vi "Spectrometer.vi"() -> ()   [LabVIEW 2018]
doc: "Demonstrates continuous waveform measurement. Spectrum is displayed in a waveform graph."
uses:
  <vilib>/Analysis/NI_AALBase.lvlib
  <vilib>/Analysis/baseanly.llb/Mean (DBL).vi
  <vilib>/Instr/_visa.llb/VISA Configure Serial Port (Instr).vi
panel:
  out "output cluster":T1={"Temperature Data"={"Bandwidth"=[10, 10, 10], "Bandwidth labels"=["Bandwidth 1-2", "Bandwidth 2-3", "Bandwidth 1-3"], "Color Temperatures"=[[nan], [nan], [nan]], "Wavelength labels"=["Temp1050-1120", "Temp1050-1230", "Temp1120-1230"], "seconds since 1Jan1904"=timestamp(3606762291.6799974 s since 1904-01-01)}, "Vis Data"={{"visible wl array"=array[2028 elements], array[2028 elements]}, {"Vis or NIR"="Visible", "Multiplexer Response"="1", "Wavelength Difference Vis (nm)"=100.0, "Vis Integration Time (ms)"=200, "Normalization path"=path "E:/Materials Testing/Calibration/2017-11-09/Multiplexter.tdms", "Vis background wave"={array[2028 elements], array[2028 elements]}}}, "NIR Data"={{"NIR wl array"=array[512 elements], array[512 elements]}, {"Vis or NIR"="NIR", "Multiplexer Response"="1", "NIR Integration Time (ms)"=50, "Wavelength Difference NIR (nm) "=100.0, "Normalization path"=path "E:/Materials Testing/Calibration/2017-11-09/Multiplexter.tdms", "NIR background wave"={array[512 elements], array[512 elements]}}}}
  out "NIR Data":T2={{"NIR wl array"=array[512 elements], array[512 elements]}, {"Vis or NIR"="NIR", "Multiplexer Response"="1", "NIR Integration Time (ms)"=50, "Wavelength Difference NIR (nm) "=100.0, "Normalization path"=path "E:/Materials Testing/Calibration/2017-11-09/Multiplexter.tdms", "NIR background wave"={array[512 elements], array[512 elements]}}}
  out "Vis Data":T3={{"visible wl array"=array[2028 elements], array[2028 elements]}, {"Vis or NIR"="Visible", "Multiplexer Response"="1", "Wavelength Difference Vis (nm)"=100.0, "Vis Integration Time (ms)"=200, "Normalization path"=path "E:/Materials Testing/Calibration/2017-11-09/Multiplexter.tdms", "Vis background wave"={array[2028 elements], array[2028 elements]}}}
  out "NIR status":bool=TRUE
  out "Vis Status":bool=TRUE
  out "file size":i64
  in  "Save NIR":bool
  in  "Save vis":bool
  in  "Tab Control 2":enum32{"Main", "Extra", "Norm", "Temperature"}(tab)
  out "Norm Visible Intensity":cluster{dbl[], dbl[]}(graph)
  out "Overload vis":bool
  out "Norm NIR Intensity":cluster{dbl[], dbl[]}(graph)
  out "Overload NIR":bool
  in  "Bandwidth 1":i32=10
  in  "Wavelength 1":dbl=1050.0 format="%#_13g"
  out "stddev":dbl=20.177756573412168
  out "Mean":dbl=-49.89258514096029 format="%0.2f"
  out "Temp 1-2":dbl=nan
  in  "Bandwidth 2":i32=10
  in  "Wavelength 2":dbl=1120.0 format="%#_13g"
  out "stddev 2":dbl=26.325405246633235
  out "Mean 2":dbl=-31.365757752015657 format="%0.2f"
  out "Temp 1-3":dbl=nan
  in  "Bandwidth 3":i32=10
  in  "Wavelength 3":dbl=1230.0 format="%#_13g"
  out "Mean 3":dbl=-15.527840110907093 format="%0.2f"
  out "stddev 3":dbl=7.686763202446039
  out "Temp 2-3":dbl=nan
  out "Visible Raw":cluster{dbl[], dbl[]}(graph)
  out "NIR Raw":cluster{dbl[], dbl[]}(graph)
  out "Subtracted NIR":cluster{dbl[], dbl[]}(graph)
  out "Subtracted Avg NIR":dbl=-353.76370072834914 format="%0.2f"
  out "Subtracted Vis":cluster{dbl[], dbl[]}(graph)
  out "Subtracted Avg Vis":dbl=-252.1229874047288 format="%0.2f"
  out "Vis norm wave":cluster{dbl[], dbl[]}(graph)
  out "NIR norm wave":cluster{dbl[], dbl[]}(graph)
  out "NIR background wave":cluster{dbl[], dbl[]}(graph)
  in  "Aquire BG vis":bool
  in  "Reset BG Vis":bool
  in  "Aquire BG NIR":bool
  in  "Reset BG NIR":bool
  out "# averages Vis":i32=10
  out "# averages NIR":i32=43
  out "Vis background wave":cluster{dbl[], dbl[]}(graph)
  in  "Wavelength Difference NIR (nm)":dbl=100.0
  out "Color Temperature NIR":cluster{"wl out":dbl[], "FT":dbl[]}(graph)={"wl out"=array[231 elements], "FT"=[nan, nan, nan, nan, nan, nan, nan, nan, nan, nan, nan, nan, nan, nan, nan, nan, nan, nan, nan, nan, nan, nan, nan, nan, nan, nan, nan, nan, nan, nan, nan, nan, nan, nan, nan, nan, nan, nan, nan, nan, nan, nan, nan, nan, nan, nan, nan, nan, nan, nan, nan, nan, nan, nan, nan, nan, nan, nan, nan, nan, nan, nan, nan, nan, nan, nan, nan, nan, nan, nan, nan, nan, nan, nan, nan, nan, nan, nan, nan, nan, nan, nan, nan, nan, nan, nan, nan, nan, nan, nan, nan, nan, nan, nan, nan, nan, nan, nan, nan, nan, nan, nan, nan, nan, nan, nan, nan, nan, nan, nan, nan, nan, nan, nan, nan, nan, nan, nan, nan, nan, nan, nan, nan, nan, nan, nan, nan, nan, nan, nan, nan, nan, nan, nan, nan, nan, nan, nan, nan, nan, nan, nan, nan, nan, nan, nan, nan, nan, nan, nan, nan, nan, nan, nan, nan, nan, nan, nan, nan, nan, nan, nan, nan, nan, nan, nan, nan, nan, nan, nan, nan, nan, nan, nan, nan, nan, nan, nan, nan, nan, nan, nan, nan, nan, nan, nan, nan, nan, nan, nan, nan, nan, nan, nan, nan, nan, nan, nan, nan, nan, nan, nan, nan, nan, nan, nan, nan, nan, nan, nan, nan, nan, nan, nan, nan, nan, nan, nan, nan, nan, nan, nan, nan, nan, nan, nan, nan, nan, nan, nan, nan]}
  in  "Wavelength Difference Vis (nm)":dbl=100.0
  out "Color Temperature Vis":cluster{"wl out":dbl[], "FT":dbl[]}(graph)
  in  "Tab Control":enum32{"Aquisition", "Setup", "File"}(tab)=enum."Setup"
  in  "Position":i32=1 min=0 max=7
  in  "Multiplexer Command":T4(ring)
  out "Multiplexer Response":string="1"
  in  "Send to multiplexer":bool
  out "NIR aq #":i32=1
  out "vis aq #":i32=1
  in  "save both":bool
  out "MP0 obtained":bool
  out "MP1 obtained":bool
  in  "Stop aquisition":bool
  in  "Multiplexer":refnum<visa-resource-name>="COM7"
  in  "NIR address":refnum<visa-resource-name>="USB0::0x2457::0x1026::NI-VISA-80002::RAW"
  in  "Visible address":refnum<visa-resource-name>="USB0::0x2457::0x101E::NI-VISA-80001::RAW"
  in  "NIR Integration Time (ms)":u32=50
  in  "Vis Integration Time (ms)":u32=200
  in  "set vis aq":i32=50
  in  "set IR aq":i32=100
  in  "Autoswitch":bool
  in  "Use NIR?":bool=TRUE
  in  "Use Vis?":bool=TRUE
  in  "Use MP":bool=TRUE
  in  "Vis every x aquisition":i32=1
  in  "NIR every x aquisition":i32=1
  in  "Mode":T5(ring)
  in  "reset aquisitions":bool
  in  "Cal params":bool
  in  "Clear":bool
  in  "Filename":string="Run1_Spectrometer"
  in  "base path":path=path "E:/Materials Testing"
  out "file path":path=path "E:/Materials Testing/2018-04-16/Run2_Spectrometer.tdms"
  in  "Normalization path":path=path "E:/Materials Testing/Calibration/2017-11-09/Multiplexter.tdms"
  out "Chg vis time":bool
  out "Change NIR time":bool
  out "tdms error out":errorcluster
  out "tdms file out":refnum<k34>
  out "visible wl array":dbl[](array[numeric])=[197.50078789145437, 197.86086398449223, 198.2209166909286, 198.58094600092215, 198.9409519046316, 199.30093439221562, 199.66089345383293, 200.02082907964217, 200.38074125980208, 200.7406299844713, 201.10049524380858, 201.46033702797257, 201.82015532712202, 202.17995013141555, 202.53972143101186, 202.89946921606966, 203.25919347674764, 203.6188942032045, 203.9785713855989, 204.33822501408957, 204.6978550788352, 205.05746156999442, 205.417044477726, 205.77660379218858, 206.13613950354087, 206.49565160194152, 206.85514007754927, 207.21460492052282, 207.5740461210208, 207.93346366920198, 208.292857555225, 208.65222776924855, 209.0115743014313, 209.370897141932, 209.73019628090933, 210.08947170852198, 210.44872341492857, 210.80795139028788, 211.16715562475855, 211.52633610849932, 211.8854928316688, 212.24462578442572, 212.6037349569288, 212.96282033933673, 213.32188192180817, 213.6809196945018, 214.03993364757636, 214.3989237711905, 214.75789005550288, 215.1168324906723, 215.47575106685738, 215.8346457742168, 216.19351660290926, 216.5523635430935, 216.91118658492812, 217.2699857185719, 217.62876093418345, 217.98751222192146, 218.34623957194475, 218.7049429744119, 219.0636224194816, 219.42227789731257, 219.78090939806347, 220.13951691189305, 220.49810042895996, 220.85665993942288, 221.21519543344058, 221.57370690117162, 221.9321943327748, 222.29065771840874, 222.6490970482322, 223.00751231240378, 223.36590350108227, 223.7242706044263, 224.08261361259454, 224.44093251574577, 224.7992273040386, 225.15749796763174, 225.5157444966839, 225.87396688135377, 226.23216511179996, 226.59033917818132, 226.9484890706564, 227.30661477938395, 227.66471629452266, 228.0227936062312, 228.38084670466833, 228.7388755799926, 229.09688022236284, 229.45486062193766, 229.81281676887576, 230.1707486533359, 230.52865626547668, 230.88653959545687, 231.24439863343508, 231.6022333695701, 231.96004379402046, 232.31782989694503, 232.6755916685024, 233.0333290988513, 233.3910421781504, 233.74873089655836, 234.10639524423397, 234.46403521133578, 234.82165078802265, 235.1792419644531, 235.53680873078594, 235.89435107717983, 236.2518689937934, 236.60936247078544, 236.9668314983146, 237.32427606653954, 237.68169616561894, 238.0390917857116, 238.3964629169761, 238.75380954957114, 239.11113167365548, 239.46842927938778, 239.82570235692668, 240.1829508964309, 240.5401748880592, 240.89737432197015, 241.25454918832256, 241.611699477275, 241.96882517898626, 242.325926283615, 242.6830027813199, 243.04005466225968, 243.39708191659298, 243.75408453447852, 244.11106250607497, 244.46801582154106, 244.82494447103548, 245.1818484447169, 245.53872773274398, 245.89558232527546, 246.25241221247003, 246.60921738448633, 246.9659978314831, 247.322753543619, 247.6794845110528, 248.03619072394306, 248.3928721724486, 248.749528846728, 249.10616073694, 249.46276783324333, 249.8193501257966, 250.17590760475855, 250.5324402602879, 250.88894808254327, 251.24543106168338, 251.60188918786693, 251.95832245125263, 252.31473084199914, 252.67111435026513, 253.02747296620936, 253.38380667999044, 253.74011548176713, 254.0963993616981, 254.45265830994202, 254.8088923166576, 255.1651013720035, 255.52128546613844, 255.87744458922117, 256.2335787314102, 256.5896878828644, 256.9457720337424, 257.3018311742029, 257.65786529440453, 258.0138743845061, 258.36985843466624, 258.7258174350435, 259.0817513757968, 259.43766024708475, 259.79354403906603, 260.1494027418993, 260.5052363457432, 260.8610448407566, 261.21682821709805, 261.57258646492625, 261.92831957439995, 262.2840275356779, 262.6397103389185, 262.99536797428084, 263.35100043192335, 263.7066077020047, 264.0621897746837, 264.41774664011905, 264.7732782884694, 265.1287847098934, 265.48426589454976, 265.8397218325972, 266.19515251419443, 266.55055792950014, 266.9059380686729, 267.2612929218716, 267.6166224792547, 267.97192673098107, 268.32720566720934, 268.68245927809824, 269.0376875538064, 269.3928904844925, 269.74806806031535, 270.1032202714335, 270.4583471080056, 270.81344856019064, 271.168524618147, 271.5235752720335, 271.87860051200875, 272.2336003282316, 272.58857471086054, 272.94352365005443, 273.29844713597197, 273.6533451587717, 274.0082177086124, 274.3630647756526, 274.71788635005134, 275.07268242196704, 275.4274529815584, 275.7821980189842, 276.1369175244032, 276.4916114879739, 276.8462798998551, 277.20092275020545, 277.5555400291837, 277.9101317269485, 278.26469783365854, 278.61923833947253, 278.9737532345491, 279.328242509047, 279.682706153125, 280.0371441569416, 280.3915565106556, 280.74594320442577, 281.1003042284106, 281.45463957276894, 281.8089492276594, 282.16323318324083, 282.51749142967174, 282.87172395711076, 283.2259307557168, 283.5801118156484, 283.9342671270643, 284.2883966801232, 284.64250046498387, 284.99657847180487, 285.3506306907448, 285.70465711196255, 286.05865772561685, 286.4126325218662, 286.7665814908693, 287.12050462278506, 287.474401907772, 287.82827333598885, 288.1821188975942, 288.53593858274684, 288.8897323816055, 289.24350028432883, 289.59724228107547, 289.95095836200414, 290.3046485172736, 290.6583127370424, 291.0119510114694, 291.36556333071314, 291.71914968493246, 292.0727100642859, 292.4262444589323, 292.7797528590301, 293.1332352547383, 293.4866916362154, 293.84012199362024, 294.1935263171113, 294.54690459684736, 294.9002568229872, 295.25358298568943, 295.6068830751127, 295.96015708141584, 296.3134049947575, 296.66662680529623, 297.0198225031908, 297.37299207859996, 297.7261355216824, 298.0792528225967, 298.43234397150167, 298.78540895855593, 299.1384477739182, 299.4914604077471, 299.8444468502015, 300.1974070914399, 300.55034112162116, 300.90324893090377, 301.2561305094466, 301.60898584740823, 301.96181493494737, 302.3146177622227, 302.66739431939305, 303.02014459661694, 303.3728685840531, 303.7255662718604, 304.0782376501972, 304.4308827092223, 304.78350143909466, 305.1360938299727, 305.48865987201515, 305.8411995553807, 306.1937128702281, 306.546199806716, 306.89866035500313, 307.25109450524815, 307.60350224760975, 307.9558835722466, 308.30823846931736, 308.6605669289809, 309.0128689413957, 309.3651444967206, 309.71739358511417, 310.06961619673524, 310.42181232174227, 310.77398195029417, 311.1261250725496, 311.4782416786672, 311.83033175880564, 312.18239530312366, 312.53443230177993, 312.88644274493316, 313.238426622742, 313.5903839253652, 313.9423146429613, 314.29421876568927, 314.64609628370755, 314.997947187175, 315.34977146625016, 315.70156911109177, 316.0533401118586, 316.4050844587093, 316.75680214180244, 317.1084931512969, 317.46015747735123, 317.8117951101242, 318.1634060397745, 318.5149902564608, 318.8665477503418, 319.21807851157615, 319.5695825303225, 319.9210597967397, 320.27251030098626, 320.623934033221, 320.9753309836027, 321.32670114228983, 321.67804449944117, 322.02936104521535, 322.3806507697712, 322.7319136632674, 323.0831497158624, 323.4343589177152, 323.7855412589844, 324.13669672982854, 324.48782532040644, 324.83892702087684, 325.1900018213983, 325.5410497121295, 325.89207068322935, 326.24306472485637, 326.5940318271692, 326.94497198032667, 327.2958851744874, 327.6467713998101, 327.9976306464534, 328.3484629045761, 328.6992681643368, 329.05004641589414, 329.400797649407, 329.75152185503396, 330.1022190229337, 330.4528891432649, 330.8035322061862, 331.1541482018565, 331.5047371204343, 331.85529895207833, 332.20583368694736, 332.5563413152, 332.9068218269949, 333.25727521249087, 333.60770146184655, 333.9581005652206, 334.3084725127717, 334.6588172946586, 335.00913490104006, 335.3594253220745, 335.7096885479209, 336.0599245687378, 336.410133374684, 336.7603149559179, 337.11046930259863, 337.4605964048846, 337.8106962529345, 338.16076883690715, 338.5108141469612, 338.8608321732553, 339.21082290594813, 339.5607863351984, 339.9107224511648, 340.26063124400605, 340.6105127038808, 340.96036682094774, 341.31019358536565, 341.6599929872931, 342.0097650168888, 342.3595096643115, 342.70922691971987, 343.05891677327253, 343.4085792151283, 343.7582142354459, 344.10782182438373, 344.4574019721008, 344.8069546687557, 345.1564799045071, 345.50597766951347, 345.85544795393395, 346.204890747927, 346.5543060416512, 346.90369382526535, 347.2530540889282, 347.60238682279845, 347.9516920170346, 348.3009696617955, 348.6502197472398, 348.99944226352625, 349.3486372008134, 349.6978045492601, 350.04694429902503, 350.3960564402667, 350.7451409631439, 351.09419785781546, 351.4432271144399, 351.7922287231759, 352.14120267418235, 352.4901489576177, 352.83906756364075, 353.18795848241024, 353.5368217040848, 353.8856572188231, 354.2344650167838, 354.5832450881258, 354.93199742300754, 355.28072201158784, 355.62941884402534, 355.9780879104788, 356.3267292011068, 356.6753427060681, 357.02392841552137, 357.3724863196254, 357.72101640853873, 358.0695186724201, 358.41799310142824, 358.7664396857219, 359.11485841545954, 359.4632492808001, 359.8116122719022, 360.15994737892447, 360.50825459202554, 360.8565339013643, 361.20478529709936, 361.5530087693893, 361.9012043083929, 362.2493719042689, 362.59751154717594, 362.9456232272726, 363.2937069347179, 363.6417626596701, 363.9897903922882, 364.3377901227308, 364.68576184115653, 365.03370553772413, 365.38162120259227, 365.72950882591977, 366.0773683978652, 366.42519990858716, 366.7730033482445, 367.1207787069959, 367.46852597500003, 367.8162451424154, 368.163936199401, 368.5115991361154, 368.85923394271725, 369.20684060936514, 369.5544191262181, 369.90196948343447, 370.249491671173, 370.5969856795926, 370.94445149885183, 371.29188911910927, 371.6392985305237, 371.9866797232539, 372.3340326874585, 372.6813574132961, 373.02865389092545, 373.3759221105053, 373.7231620621942, 374.070373736151, 374.4175571225344, 374.76471221150297, 375.1118389932154, 375.4589374578304, 375.8060075955068, 376.1530493964031, 376.50006285067803, 376.84704794849046, 377.1940046799989, 377.54093303536206, 377.8878330047386, 378.23470457828734, 378.58154774616685, 378.92836249853576, 379.27514882555306, 379.62190671737716, 379.96863616416687, 380.3153371560808, 380.66200968327774, 381.00865373591637, 381.3552693041552, 381.7018563781531, 382.0484149480688, 382.39494500406084, 382.74144653628804, 383.087919534909, 383.4343639900825, 383.7807798919671, 384.1271672307216, 384.4735259965047, 384.819856179475, 385.1661577697912, 385.5124307576121, 385.85867513309637, 386.20489088640255, 386.5510780076894, 386.8972364871158, 387.24336631484016, 387.5894674810213, 387.93553997581796, 388.2815837893888, 388.62759891189245, 388.97358533348756, 389.31954304433305, 389.66547203458737, 390.0113722944093, 390.35724381395755, 390.7030865833908, 391.04890059286777, 391.394685832547, 391.74044229258743, 392.08616996314754, 392.431868834386, 392.77753889646175, 393.12318013953336, 393.4687925537594, 393.8143761292986, 394.1599308563098, 394.5054567249516, 394.85095372538257, 395.19642184776154, 395.5418610822473, 395.8872714189983, 396.23265284817336, 396.5780053599312, 396.9233289444304, 397.2686235918298, 397.6138892922879, 397.9591260359636, 398.3043338130155, 398.64951261360216, 398.99466242788253, 399.3397832460151, 399.6848750581586, 400.0299378544717, 400.3749716251133, 400.71997636024184, 401.064952050016, 401.4098986845947, 401.7548162541365, 402.0997047488, 402.44456415874396, 402.7893944741272, 403.1341956851083, 403.4789677818458, 403.8237107544987, 404.1684245932255, 404.5131092881849, 404.8577648295356, 405.2023912074364, 405.54698841204583, 405.8915564335226, 406.23609526202546, 406.58060488771315, 406.9250853007443, 407.2695364912775, 407.6139584494717, 407.95835116548534, 408.30271462947724, 408.64704883160596, 408.99135376203037, 409.33562941090906, 409.6798757684007, 410.0240928246641, 410.36828056985786, 410.7124389941406, 411.0565680876711, 411.40066784060815, 411.74473824311025, 412.0887792853361, 412.4327909574446, 412.77677324959427, 413.12072615194376, 413.46464965465185, 413.8085437478773, 414.1524084217787, 414.49624366651466, 414.84004947224406, 415.18382582912545, 415.5275727273176, 415.87129015697917, 416.2149781082689, 416.5586365713454, 416.90226553636734, 417.24586499349346, 417.5894349328825, 417.9329753446931, 418.27648621908395, 418.6199675462138, 418.96341931624124, 419.306841519325, 419.65023414562376, 419.99359718529627, 420.3369306285012, 420.6802344653972, 421.023508686143, 421.3667532808972, 421.70996823981864, 422.0531535530659, 422.3963092107977, 422.73943520317283, 423.08253152034973, 423.4255981524874, 423.76863508974435, 424.1116423222792, 424.4546198402508, 424.7975676338178, 425.1404856931389, 425.4833740083726, 425.8262325696779, 426.16906136721343, 426.51186039113765, 426.8546296316094, 427.19736907878746, 427.5400787228304, 427.88275855389685, 428.2254085621457, 428.56802873773546, 428.9106190708249, 429.2531795515727, 429.5957101701376, 429.9382109166782, 430.2806817813532, 430.6231227543214, 430.96553382574143, 431.3079149857719, 431.65026622457157, 431.9925875322992, 432.3348788991134, 432.6771403151728, 433.01937177063616, 433.3615732556622, 433.7037447604096, 434.045886275037, 434.3879977897032, 434.7300792945668, 435.07213077978645, 435.4141522355209, 435.7561436519289, 436.098105019169, 436.4400363273999, 436.7819375667805, 437.1238087274694, 437.4656497996251, 437.80746077340643, 438.1492416389722, 438.49099238648097, 438.8327130060914, 439.17440348796214, 439.5160638222521, 439.85769399911976, 440.19929400872394, 440.54086384122326, 440.88240348677647, 441.22391293554205, 441.5653921776791, 441.90684120334595, 442.24826000270144, 442.5896485659041, 442.93100688311296, 443.2723349444864, 443.6136327401831, 443.9549002603621, 444.29613749518177, 444.6373444348009, 444.9785210693781, 445.3196673890722, 445.6607833840418, 446.0018690444455, 446.3429243604423, 446.6839493221906, 447.0249439198492, 447.3659081435767, 447.70684198353194, 448.04774542987354, 448.3886184727602, 448.7294611023505, 449.07027330880334, 449.4110550822773, 449.7518064129309, 450.09252729092316, 450.4332177064126, 450.77387764955796, 451.11450711051776, 451.4551060794509, 451.79567454651607, 452.1362125018717, 452.4767199356768, 452.81719683808996, 453.1576431992698, 453.49805900937497, 453.8384442585643, 454.1787989369965, 454.51912303483, 454.8594165422238, 455.19967944933643, 455.53991174632665, 455.88011342335307, 456.2202844705745, 456.5604248781495, 456.9005346362367, 457.24061373499507, 457.58066216458315, 457.9206799151596, 458.260666976883, 458.6006233399123, 458.9405489944061, 459.280443930523, 459.62030813842165, 459.96014160826087, 460.2999443301994, 460.6397162943957, 460.97945749100876, 461.3191679101971, 461.6588475421194, 461.9984963769343, 462.3381144048007, 462.67770161587714, 463.0172580003222, 463.35678354829486, 463.6962782499536, 464.0357420954572, 464.37517507496415, 464.7145771786335, 465.05394839662364, 465.39328871909333, 465.73259813620143, 466.07187663810646, 466.4111242149671, 466.75034085694205, 467.0895265541902, 467.42868129686997, 467.76780507514013, 468.1068978791595, 468.44595969908664, 468.7849905250803, 469.12399034729907, 469.46295915590173, 469.80189694104706, 470.1408036928936, 470.4796794015999, 470.8185240573251, 471.1573376502276, 471.49612017046593, 471.83487160819914, 472.17359195358574, 472.5122811967844, 472.8509393279538, 473.18956633725276, 473.5281622148398, 473.8667269508738, 474.2052605355132, 474.54376295891706, 474.8822342112437, 475.2206742826519, 475.55908316330056, 475.8974608433482, 476.2358073129534, 476.5741225622751, 476.9124065814719, 477.25065936070246, 477.5888808901253, 477.92707115989947, 478.2652301601835, 478.6033578811358, 478.9414543129156, 479.2795194456812, 479.61755326959144, 479.9555557748049, 480.2935269514804, 480.6314667897766, 480.96937527985216, 481.30725241186565, 481.64509817597605, 481.9829125623418, 482.3206955611216, 482.6584471624743, 482.9961673565586, 483.333856133533, 483.6715134835562, 484.0091393967872, 484.3467338633844, 484.68429687350636, 485.02182841731224, 485.3593284849603, 485.6967970666096, 486.0342341524184, 486.37163973254565, 486.7090137971501, 487.04635633639026, 487.38366734042495, 487.72094679941284, 488.05819470351264, 488.39541104288287, 488.73259580768246, 489.06974898807, 489.40687057420405, 489.7439605562435, 490.08101892434706, 490.41804566867324, 490.75504077938075, 491.09200424662845, 491.4289360605749, 491.7658362113788, 492.1027046891989, 492.4395414841938, 492.7763465865223, 493.11311998634295, 493.44986167381455, 493.7865716390959, 494.1232498723454, 494.4598963637219, 494.79651110338415, 495.1330940814908, 495.46964528820035, 495.8061647136718, 496.1426523480638, 496.4791081815348, 496.8155322042436, 497.151924406349, 497.4882847780096, 497.824613309384, 498.1609099906312, 498.49717481190953, 498.833407763378, 499.1696088351949, 499.5057780175193, 499.8419153005097, 500.1780206743248, 500.51409412912346, 500.85013565506415, 501.18614524230577, 501.5221228810067, 501.8580685613259, 502.1939822734221, 502.5298640074538, 502.8657137535797, 503.20153150195864, 503.5373172427492, 503.87307096611, 504.2087926622, 504.54448232117767, 504.88013993320175, 505.2157654884308, 505.5513589770238, 505.8869203891392, 506.22244971493575, 506.5579469445723, 506.8934120682073, 507.2288450759996, 507.56424595810773, 507.8996147046906, 508.2349513059068, 508.5702557519149, 508.9055280328738, 509.24076813894203, 509.57597606027844, 509.91115178704143, 510.2462953093901, 510.5814066174828, 510.91648570147834, 511.25153255153543, 511.5865471578128, 511.9215295104691, 512.256479599663, 512.591397415553, 512.9262829482982, 513.2611361880572, 513.5959571249882, 513.9307457492506, 514.2655020510026, 514.6002260204029, 514.9349176476106, 515.269576922784, 515.604203836082, 515.9387983776631, 516.2733605376862, 516.6078903063099, 516.9423876736927, 517.2768526299936, 517.6112851653712, 517.9456852699841, 518.280052933991, 518.6143881475507, 518.9486909008219, 519.2829611839629, 519.6171989871331, 519.9514043004906, 520.2855771141943, 520.6197174184027, 520.953825203275, 521.2879004589694, 521.6219431756447, 521.9559533434598, 522.2899309525732, 522.6238759931435, 522.9577884553295, 523.29166832929, 523.6255156051835, 523.959330273169, 524.2931123234048, 524.6268617460498, 524.9605785312627, 525.294262669202, 525.6279141500266, 525.9615329638953, 526.2951191009665, 526.6286725513991, 526.9621933053515, 527.2956813529828, 527.6291366844514, 527.962559289916, 528.2959491595356, 528.6293062834684, 528.9626306518735, 529.2959222549093, 529.6291810827348, 529.9624071255084, 530.295600373389, 530.6287608165352, 530.9618884451056, 531.294983249259, 531.628045219154, 531.9610743449496, 532.2940706168041, 532.6270340248764, 532.9599645593252, 533.2928622103091, 533.6257269679866, 533.9585588225167, 534.2913577640583, 534.6241237827694, 534.9568568688093, 535.2895570123364, 535.6222242035095, 535.9548584324872, 536.2874596894284, 536.6200279644914, 536.9525632478354, 537.2850655296186, 537.6175347999999, 537.9499710491383, 538.2823742671917, 538.6147444443196, 538.9470815706804, 539.2793856364327, 539.6116566317352, 539.9438945467468, 540.2760993716258, 540.6082710965313, 540.9404097116218, 541.2725152070559, 541.6045875729926, 541.9366267995902, 542.2686328770076, 542.6006057954036, 542.9325455449366, 543.2644521157656, 543.596325498049, 543.9281656819459, 544.2599726576144, 544.5917464152136, 544.9234869449022, 545.2551942368387, 545.5868682811819, 545.9185090680907, 546.2501165877233, 546.5816908302387, 546.9132317857957, 547.2447394445527, 547.5762137966686, 547.9076548323019, 548.2390625416117, 548.5704369147561, 548.9017779418941, 549.2330856131847, 549.5643599187861, 549.8956008488572, 550.2268083935564, 550.557982543043, 550.8891232874752, 551.2202306170118, 551.5513045218116, 551.8823449920332, 552.2133520178353, 552.5443255893765, 552.8752656968156, 553.2061723303113, 553.5370454800224, 553.8678851361074, 554.198691288725, 554.5294639280339, 554.8602030441929, 555.1909086273606, 555.5215806676957, 555.8522191553569, 556.182824080503, 556.5133954332924, 556.8439332038841, 557.1744373824366, 557.5049079591088, 557.8353449240591, 558.1657482674464, 558.4961179794293, 558.8264540501665, 559.1567564698169, 559.4870252285388, 559.8172603164911, 560.1474617238325, 560.4776294407218, 560.8077634573174, 561.1378637637782, 561.4679303502629, 561.79796320693, 562.1279623239385, 562.4579276914469, 562.7878592996138, 563.117757138598, 563.4476211985583, 563.7774514696533, 564.1072479420415, 564.4370106058819, 564.766739451333, 565.0964344685538, 565.4260956477024, 565.7557229789379, 566.085316452419, 566.4148760583043, 566.7444017867523, 567.0738936279222, 567.4033515719722, 567.7327756090612, 568.0621657293478, 568.3915219229909, 568.720844180149, 569.0501324909808, 569.3793868456451, 569.7086072343004, 570.0377936471054, 570.3669460742192, 570.6960645058, 571.0251489320068, 571.354199342998, 571.6832157289325, 572.012198079969, 572.3411463862662, 572.6700606379826, 572.9989408252771, 573.3277869383085, 573.656598967235, 573.9853769022158, 574.3141207334094, 574.6428304509742, 574.9715060450694, 575.3001475058535, 575.6287548234851, 575.9573279881229, 576.2858669899257, 576.614371819052, 576.9428424656608, 577.2712789199104, 577.5996811719598, 577.9280492119675, 578.2563830300924, 578.5846826164931, 578.9129479613282, 579.2411790547563, 579.5693758869364, 579.897538448027, 580.2256667281869, 580.5537607175745, 580.881820406349, 581.2098457846686, 581.5378368426922, 581.8657935705785, 582.1937159584861, 582.5216039965738, 582.8494576750003, 583.1772769839243, 583.5050619135044, 583.8328124538992, 584.1605285952676, 584.4882103277681, 584.8158576415597, 585.1434705268006, 585.47104897365, 585.7985929722663, 586.1261025128083, 586.4535775854345, 586.7810181803039, 587.108424287575, 587.4357958974065, 587.7631329999571, 588.0904355853854, 588.4177036438505, 588.7449371655104, 589.0721361405243, 589.399300559051, 589.7264304112487, 590.0535256872763, 590.3805863772927, 590.7076124714565, 591.0346039599261, 591.3615608328606, 591.6884830804185, 592.0153706927583, 592.3422236600389, 592.6690419724191, 592.9958256200574, 593.3225745931126, 593.6492888817434, 593.9759684761084, 594.3026133663662, 594.6292235426757, 594.9557989951956, 595.2823397140844, 595.6088456895009, 595.9353169116038, 596.2617533705517, 596.5881550565035, 596.9145219596176, 597.2408540700529, 597.567151377968, 597.8934138735217, 598.2196415468726, 598.5458343881794, 598.8719923876008, 599.1981155352954, 599.5242038214222, 599.8502572361394, 600.1762757696063, 600.502259411981, 600.8282081534223, 601.1541219840893, 601.4800008941403, 601.8058448737343, 602.1316539130297, 602.4574280021853, 602.7831671313596, 603.1088712907117, 603.4345404704001, 603.7601746605832, 604.0857738514202, 604.4113380330695, 604.7368671956897, 605.0623613294396, 605.3878204244782, 605.7132444709637, 606.038633459055, 606.3639873789108, 606.6893062206898, 607.0145899745506, 607.3398386306519, 607.6650521791527, 607.9902306102114, 608.3153739139866, 608.6404820806371, 608.9655551003217, 609.290592963199, 609.6155956594275, 609.9405631791664, 610.2654955125739, 610.590392649809, 610.91525458103, 611.240081296396, 611.5648727860656, 611.8896290401973, 612.2143500489501, 612.5390358024824, 612.8636862909531, 613.1883015045205, 613.5128814333439, 613.8374260675815, 614.1619353973922, 614.4864094129347, 614.8108481043677, 615.1352514618497, 615.4596194755395, 615.783952135596, 616.1082494321777, 616.4325113554431, 616.7567378955513, 617.0809290426607, 617.40508478693, 617.729205118518, 618.0532900275834, 618.3773395042849, 618.7013535387812, 619.0253321212307, 619.3492752417924, 619.673182890625, 619.997055057887, 620.3208917337372, 620.6446929083343, 620.9684585718371, 621.2921887144039, 621.6158833261939, 621.9395423973655, 622.2631659180772, 622.5867538784881, 622.9103062687568, 623.2338230790418, 623.557304299502, 623.8807499202958, 624.2041599315822, 624.5275343235198, 624.8508730862671, 625.1741762099832, 625.4974436848265, 625.8206755009555, 626.1438716485294, 626.4670321177065, 626.7901568986455, 627.1132459815053, 627.4362993564446, 627.7593170136219, 628.0822989431958, 628.4052451353255, 628.7281555801691, 629.0510302678856, 629.3738691886335, 629.6966723325719, 630.019439689859, 630.3421712506537, 630.6648670051148, 630.9875269434009, 631.3101510556708, 631.6327393320827, 631.9552917627958, 632.2778083379688, 632.6002890477602, 632.9227338823287, 633.2451428318329, 633.5675158864319, 633.8898530362837, 634.2121542715477, 634.5344195823824, 634.856648958946, 635.1788423913978, 635.5009998698962, 635.8231213846001, 636.1452069256677, 636.4672564832583, 636.7892700475303, 637.1112476086423, 637.4331891567532, 637.7550946820215, 638.0769641746062, 638.3987976246655, 638.7205950223585, 639.0423563578438, 639.36408162128, 639.6857708028258, 640.00742389264, 640.3290408808813, 640.650621757708, 640.9721665132793, 641.2936751377538, 641.6151476212899, 641.9365839540466, 642.2579841261824, 642.5793481278561, 642.9006759492262, 643.2219675804517, 643.5432230116911, 643.8644422331031, 644.1856252348464, 644.5067720070798, 644.8278825399617, 645.1489568236511, 645.4699948483066, 645.7909966040868, 646.1119620811505, 646.4328912696564, 646.753784159763, 647.0746407416292, 647.3954610054135, 647.7162449412748, 648.0369925393718, 648.357703789863, 648.6783786829071, 648.999017208663, 649.3196193572893, 649.6401851189446, 649.9607144837876, 650.281207441977, 650.6016639836716, 650.92208409903, 651.2424677782109, 651.562815011373, 651.883125788675, 652.2034001002755, 652.5236379363333, 652.8438392870072, 653.1640041424556, 653.4841324928374, 653.8042243283113, 654.124279639036, 654.4442984151698, 654.7642806468718, 655.0842263243009, 655.4041354376151, 655.7240079769737, 656.0438439325351, 656.3636432944581, 656.6834060529012, 657.0031321980235, 657.3228217199833, 657.6424746089393, 657.9620908550505, 658.2816704484753, 658.6012133793727, 658.9207196379009, 659.240189214219, 659.5596220984856, 659.8790182808594, 660.1983777514988, 660.517700500563, 660.8369865182104, 661.1562357945996, 661.4754483198896, 661.7946240842388, 662.113763077806, 662.4328652907498, 662.7519307132291, 663.0709593354024, 663.3899511474284, 663.708906139466, 664.0278243016737, 664.3467056242102, 664.6655500972341, 664.9843577109044, 665.3031284553796, 665.6218623208182, 665.9405592973792, 666.2592193752213, 666.5778425445029, 666.8964287953828, 667.21497811802, 667.5334905025728, 667.8519659391999, 668.1704044180602, 668.4888059293124, 668.8071704631152, 669.1254980096269, 669.4437885590067, 669.762042101413, 670.0802586270046, 670.3984381259401, 670.7165805883783, 671.0346860044777, 671.3527543643974, 671.6707856582956, 671.9887798763313, 672.306737008663, 672.6246570454496, 672.9425399768495, 673.2603857930219, 673.5781944841249, 673.8959660403175, 674.2137004517583, 674.5313977086062, 674.8490578010196, 675.1666807191574, 675.4842664531782, 675.8018149932406, 676.1193263295035, 676.4368004521255, 676.754237351265, 677.0716370170811, 677.3889994397325, 677.7063246093777, 678.0236125161754, 678.3408631502843, 678.6580765018632, 678.9752525610705, 679.2923913180654, 679.6094927630062, 679.9265568860516, 680.2435836773602, 680.5605731270912, 680.8775252254028, 681.1944399624538, 681.5113173284029, 681.828157313409, 682.1449599076304, 682.4617251012262, 682.7784528843548, 683.095143247175, 683.4117961798455, 683.7284116725249, 684.044989715372, 684.3615302985455, 684.678033412204, 684.9944990465062, 685.310927191611, 685.6273178376766, 685.9436709748622, 686.2599865933264, 686.5762646832277, 686.8925052347247, 687.2087082379765, 687.5248736831414, 687.8410015603783, 688.1570918598459, 688.4731445717027, 688.7891596861077, 689.1051371932192, 689.4210770831963, 689.7369793461975, 690.0528439723814, 690.3686709519068, 690.6844602749322, 691.0002119316166, 691.3159259121186, 691.6316022065969, 691.94724080521, 692.2628416981167, 692.5784048754757, 692.8939303274458, 693.2094180441857, 693.5248680158536, 693.840280232609, 694.1556546846099, 694.4709913620153, 694.7862902549839, 695.1015513536743, 695.4167746482453, 695.7319601288555, 696.0471077856635, 696.3622176088281, 696.6772895885082, 696.9923237148621, 697.3073199780488, 697.6222783682267, 697.9371988755547, 698.2520814901915, 698.5669262022958, 698.8817330020261, 699.1965018795412, 699.511232825, 699.8259258285608, 700.1405808803826, 700.4551979706239, 700.7697770894436, 701.0843182270003, 701.3988213734524, 701.713286518959, 702.0277136536786, 702.34210276777, 702.6564538513917, 702.9707668947027, 703.2850418878613, 703.5992788210265, 703.9134776843567, 704.227638468011, 704.5417611621478, 704.8558457569258, 705.1698922425038, 705.4839006090403, 705.7978708466943, 706.1118029456243, 706.425696895989, 706.7395526879471, 707.0533703116571, 707.367149757278, 707.6808910149686, 707.9945940748871, 708.3082589271924, 708.6218855620434, 708.9354739695985, 709.2490241400166, 709.5625360634564, 709.8760097300764, 710.1894451300354, 710.5028422534921, 710.8162010906052, 711.1295216315334, 711.4428038664353, 711.7560477854696, 712.0692533787951, 712.3824206365706, 712.6955495489543, 713.0086401061054, 713.3216922981825, 713.6347061153439, 713.9476815477489, 714.2606185855557, 714.5735172189233, 714.8863774380101, 715.1991992329749, 715.5119825939765, 715.8247275111737, 716.1374339747248, 716.4501019747889, 716.7627315015244, 717.0753225450901, 717.3878750956447, 717.7003891433469, 718.0128646783554, 718.3253016908287, 718.6377001709259, 718.9500601088051, 719.2623814946255, 719.5746643185457, 719.8869085707242, 720.19911424132, 720.5112813204913, 720.8234097983973, 721.1354996651963, 721.4475509110473, 721.7595635261089, 722.0715375005396, 722.3834728244983, 722.6953694881436, 723.0072274816343, 723.319046795129, 723.6308274187863, 723.9425693427651, 724.2542725572239, 724.5659370523216, 724.8775628182166, 725.1891498450678, 725.500698123034, 725.8122076422735, 726.1236783929453, 726.4351103652082, 726.7465035492206, 727.0578579351411, 727.3691735131288, 727.6804502733422, 727.9916882059399, 728.3028873010805, 728.6140475489232, 728.9251689396261, 729.2362514633481, 729.5472951102481, 729.8582998704846, 730.1692657342163, 730.4801926916018, 730.7910807328, 731.1019298479694, 731.4127400272687, 731.7235112608569, 732.0342435388923, 732.3449368515337, 732.6555911889399, 732.9662065412695, 733.2767828986813, 733.5873202513337, 733.8978185893857, 734.208277902996, 734.5186981823231, 734.8290794175257, 735.1394215987626, 735.4497247161926, 735.759988759974, 736.0702137202659, 736.3803995872267, 736.6905463510154, 737.0006540017903, 737.3107225297105, 737.6207519249343, 737.9307421776207, 738.2406932779282, 738.5506052160156, 738.8604779820415, 739.1703115661646, 739.4801059585438, 739.7898611493374, 740.0995771287046, 740.4092538868035, 740.7188914137934, 741.0284896998324, 741.3380487350796, 741.6475685096935, 741.9570490138331, 742.2664902376567, 742.575892171323, 742.885254804991, 743.1945781288192, 743.5038621329661, 743.8131068075909, 744.1223121428519, 744.4314781289079, 744.7406047559174, 745.0496920140395, 745.3587398934326, 745.6677483842552, 745.9767174766665, 746.285647160825, 746.5945374268891, 746.9033882650178, 747.2121996653698, 747.5209716181035, 747.8297041133779, 748.1383971413516, 748.4470506921832, 748.7556647560315, 749.0642393230551, 749.3727743834128, 749.6812699272632, 749.9897259447649, 750.2981424260768, 750.6065193613575, 750.9148567407659, 751.22315455446, 751.5314127925994, 751.8396314453422, 752.1478105028474, 752.4559499552732, 752.7640497927789, 753.0721100055231, 753.3801305836639, 753.6881115173607, 753.9960527967718, 754.3039544120561, 754.611816353372, 754.9196386108785, 755.2274211747341, 755.5351640350976, 755.8428671821276, 756.1505306059828, 756.458154296822, 756.7657382448037, 757.0732824400868, 757.38078687283, 757.6882515331918, 757.9956764113309, 758.3030614974061, 758.6104067815762, 758.9177122539995, 759.2249779048351, 759.5322037242416, 759.8393897023775, 760.1465358294016, 760.4536420954728, 760.7607084907495, 761.0677350053904, 761.3747216295543, 761.6816683533999, 761.988575167086, 762.2954420607709, 762.6022690246136, 762.909056048773, 763.2158031234071, 763.5225102386753, 763.8291773847359, 764.1358045517478, 764.4423917298694, 764.7489389092598, 765.0554460800773, 765.3619132324808, 765.668340356629, 765.9747274426805, 766.281074480794, 766.5873814611282, 766.893648373842, 767.1998752090938, 767.5060619570423, 767.8122086078463, 768.1183151516645, 768.4243815786557, 768.7304078789783, 769.0363940427911, 769.3423400602532, 769.6482459215226, 769.9541116167584, 770.2599371361191, 770.5657224697637, 770.8714676078505, 771.1771725405385, 771.4828372579864, 771.7884617503526, 772.0940460077959, 772.3995900204751, 772.705093778549, 773.0105572721759, 773.3159804915148, 773.6213634267243, 773.9267060679632, 774.2320084053899, 774.5372704291634, 774.8424921294423, 775.1476734963853, 775.4528145201509, 775.7579151908982, 776.0629754987855, 776.3679954339715, 776.672974986615, 776.9779141468749, 777.2828129049097, 777.587671250878, 777.8924891749386, 778.1972666672502, 778.5020037179714, 778.806700317261, 779.1113564552777, 779.41597212218, 779.7205473081268, 780.0250820032768, 780.3295761977885, 780.6340298818207, 780.9384430455322, 781.2428156790813, 781.5471477726272, 781.8514393163284, 782.1556903003434, 782.4599007148312, 782.7640705499502, 783.0681997958593, 783.3722884427171, 783.6763364806824, 783.9803438999136, 784.2843106905698, 784.5882368428094, 784.892122346791, 785.1959671926736, 785.4997713706158, 785.8035348707763, 786.1072576833136, 786.4109397983865, 786.7145812061538, 787.0181818967741, 787.321741860406, 787.6252610872084, 787.9287395673399, 788.2321772909589, 788.5355742482247, 788.8389304292955, 789.1422458243302, 789.4455204234872, 789.7487542169257, 790.051947194804, 790.355099347281, 790.6582106645152, 790.9612811366654, 791.2643107538904, 791.5672995063485, 791.8702473841989, 792.1731543776, 792.4760204767103, 792.778845671689, 793.0816299526946, 793.3843733098855, 793.6870757334207, 793.9897372134587, 794.2923577401584, 794.5949373036783, 794.8974758941772, 795.1999735018138, 795.5024301167467, 795.8048457291346, 796.1072203291362, 796.4095539069104, 796.7118464526155, 797.0140979564105, 797.316308408454, 797.6184777989047, 797.9206061179212, 798.2226933556623, 798.5247395022868, 798.8267445479531, 799.12870848282, 799.4306312970463, 799.7325129807906, 800.0343535242115, 800.336152917468, 800.6379111507184, 800.9396282141219, 801.2413040978365, 801.5429387920215, 801.8445322868353, 802.1460845724366, 802.447595638984, 802.7490654766367, 803.0504940755528, 803.3518814258912, 803.6532275178106, 803.9545323414696, 804.2557958870271, 804.5570181446417, 804.8581991044721, 805.1593387566768, 805.4604370914146, 805.7614940988444, 806.0625097691247, 806.3634840924143, 806.6644170588717, 806.9653086586557, 807.266158881925, 807.5669677188381, 807.8677351595542, 808.1684611942316, 808.4691458130288, 808.7697890061049, 809.0703907636184, 809.3709510757282, 809.6714699325926, 809.9719473243706, 810.2723832412207, 810.5727776733019, 810.8731306107724, 811.1734420437914, 811.4737119625173, 811.7739403571087, 812.0741272177246, 812.3742725345235, 812.6743762976643, 812.9744384973052, 813.2744591236053, 813.5744381667233, 813.8743756168177, 814.1742714640474, 814.4741256985708, 814.7739383105468, 815.073709290134, 815.3734386274914, 815.6731263127772, 815.9727723361505, 816.2723766877696, 816.5719393577934, 816.8714603363808, 817.17093961369, 817.4703771798802, 817.7697730251099, 818.0691271395377, 818.3684395133223, 818.6677101366224, 818.9669389995969, 819.2661260924041, 819.565271405203, 819.8643749281524, 820.1634366514105, 820.4624565651363, 820.7614346594887, 821.0603709246261, 821.3592653507071, 821.6581179278908, 821.9569286463354, 822.2556974962, 822.5544244676429, 822.8531095508232, 823.1517527358993, 823.45035401303, 823.7489133723742, 824.0474308040901, 824.3459062983369, 824.6443398452728, 824.942731435057, 825.2410810578477, 825.539388703804, 825.8376543630843, 826.1358780258474, 826.4340596822522, 826.732199322457, 827.0302969366207, 827.328352514902, 827.6263660474597, 827.9243375244522, 828.2222669360383, 828.5201542723769, 828.8179995236263, 829.1158026799457, 829.4135637314934, 829.7112826684282, 830.0089594809086, 830.3065941590936, 830.6041866931419, 830.9017370732118, 831.1992452894625, 831.4967113320524, 831.7941351911403, 832.0915168568846, 832.3888563194444, 832.6861535689782, 832.9834085956446, 833.2806213896024, 833.5777919410103, 833.874920240027, 834.1720062768111, 834.4690500415214, 834.7660515243166, 835.0630107153553, 835.3599276047961, 835.656802182798, 835.9536344395194, 836.2504243651191, 836.5471719497558, 836.8438771835882, 837.140540056775, 837.4371605594747, 837.7337386818464, 838.0302744140483, 838.3267677462394, 838.6232186685784, 838.919627171224, 839.2159932443346, 839.5123168780691, 839.8085980625863, 840.1048367880447, 840.4010330446031, 840.6971868224201, 840.9932981116547, 841.2893669024651, 841.5853931850103, 841.8813769494488, 842.1773181859396, 842.473216884641, 842.7690730357122, 843.0648866293113, 843.3606576555975, 843.6563861047291, 843.9520719668649, 844.247715232164, 844.5433158907844, 844.8388739328851, 845.1343893486251, 845.4298621281625, 845.7252922616564, 846.0206797392655, 846.3160245511484, 846.6113266874638, 846.9065861383701, 847.2018028940264, 847.4969769445914, 847.7921082802234, 848.0871968910815, 848.3822427673242, 848.6772458991103, 848.9722062765981, 849.2671238899468, 849.5619987293148, 849.8568307848609, 850.1516200467439, 850.4463665051222, 850.7410701501547, 851.035730972, 851.3303489608169, 851.624924106764, 851.9194564, 852.2139458306835, 852.5083923889734, 852.8027960650282, 853.0971568490068, 853.3914747310677, 853.6857497013696, 853.9799817500714, 854.2741708673313, 854.5683170433086, 854.8624202681618, 855.1564805320493, 855.45049782513, 855.7444721375629, 856.0384034595061, 856.3322917811184, 856.626137092559, 856.9199393839862, 857.2136986455585, 857.5074148674352, 857.8010880397744, 858.094718152735, 858.3883051964757, 858.6818491611554, 858.9753500369324, 859.2688078139655, 859.5622224824136, 859.8555940324353, 860.1489224541893, 860.4422077378341, 860.7354498735285, 861.0286488514313, 861.3218046617011, 861.6149172944966, 861.9079867399766, 862.2010129882997, 862.4939960296243, 862.7869358541096, 863.0798324519142, 863.3726858131964, 863.6654959281152, 863.9582627868292, 864.2509863794972, 864.5436666962777, 864.8363037273297, 865.1288974628114, 865.421447892882, 865.7139550077]
  out "NIR wl array":dbl[](array[numeric])=[890.92688, 894.2151612831569, 897.503264932628, 900.7911909484129, 904.0789393305121, 907.366510078925, 910.653903193652, 913.941118674693, 917.2281565220479, 920.515016735717, 923.8016993156999, 927.088204261997, 930.374531574608, 933.660681253533, 936.9466532987719, 940.2324477103249, 943.518064488192, 946.803503632373, 950.088765142868, 953.373849019677, 956.6587552627999, 959.943483872237, 963.2280348479879, 966.5124081900531, 969.796603898432, 973.0806219731251, 976.3644624141319, 979.6481252214529, 982.931610395088, 986.214917935037, 989.4980478413, 992.781000113877, 996.063774752768, 999.346371757973, 1002.6287911294919, 1005.911032867325, 1009.193096971472, 1012.474983441933, 1015.756692278708, 1019.038223481797, 1022.3195770512, 1025.6007529869169, 1028.881751288948, 1032.162571957293, 1035.443214991952, 1038.723680392925, 1042.003968160212, 1045.2840782938129, 1048.564010793728, 1051.843765659957, 1055.1233428925, 1058.402742491357, 1061.681964456528, 1064.961008788013, 1068.2398754858118, 1071.518564549925, 1074.797075980352, 1078.075409777093, 1081.353565940148, 1084.631544469517, 1087.9093453652001, 1091.1869686271968, 1094.464414255508, 1097.741682250133, 1101.018772611072, 1104.295685338325, 1107.572420431892, 1110.848977891773, 1114.125357717968, 1117.4015599104769, 1120.6775844693, 1123.953431394437, 1127.229100685888, 1130.504592343653, 1133.779906367732, 1137.055042758125, 1140.330001514832, 1143.604782637853, 1146.8793861271881, 1150.153811982837, 1153.4280602048, 1156.7021307930768, 1159.9760237476678, 1163.249739068573, 1166.523276755792, 1169.796636809325, 1173.069819229172, 1176.342824015333, 1179.6156511678078, 1182.888300686597, 1186.1607725717, 1189.433066823117, 1192.705183440848, 1195.977122424893, 1199.248883775252, 1202.5204674919248, 1205.791873574912, 1209.0631020242129, 1212.334152839828, 1215.605026021757, 1218.87572157, 1222.146239484557, 1225.4165797654277, 1228.6867424126128, 1231.956727426112, 1235.226534805925, 1238.4961645520518, 1241.7656166644929, 1245.034891143248, 1248.3039879883167, 1251.5729071997, 1254.841648777397, 1258.110212721408, 1261.3785990317328, 1264.6468077083719, 1267.914838751325, 1271.1826921605918, 1274.4503679361728, 1277.717866078068, 1280.985186586277, 1284.2523294608, 1287.519294701637, 1290.786082308788, 1294.0526922822528, 1297.319124622032, 1300.585379328125, 1303.851456400532, 1307.117355839253, 1310.383077644288, 1313.648621815637, 1316.9139883532998, 1320.179177257277, 1323.444188527568, 1326.7090221641731, 1329.973678167092, 1333.238156536325, 1336.5024572718721, 1339.766580373733, 1343.030525841908, 1346.294293676397, 1349.5578838772, 1352.8212964443169, 1356.084531377748, 1359.3475886774931, 1362.610468343552, 1365.873170375925, 1369.135694774612, 1372.3980415396131, 1375.6602106709279, 1378.922202168557, 1382.1840160325, 1385.445652262757, 1388.707110859328, 1391.968391822213, 1395.229495151412, 1398.490420846925, 1401.7511689087519, 1405.0117393368928, 1408.272132131348, 1411.532347292117, 1414.7923848192, 1418.052244712597, 1421.311926972308, 1424.571431598333, 1427.8307585906718, 1431.089907949325, 1434.348879674292, 1437.607673765573, 1440.866290223168, 1444.124729047077, 1447.3829902373, 1450.6410737938368, 1453.8989797166878, 1457.156708005853, 1460.414258661332, 1463.671631683125, 1466.928827071232, 1470.185844825653, 1473.4426849463878, 1476.699347433437, 1479.9558322868, 1483.2121395064771, 1486.468269092468, 1489.724221044773, 1492.979995363392, 1496.2355920483249, 1499.491011099572, 1502.746252517133, 1506.001316301008, 1509.2562024511972, 1512.5109109676998, 1515.765441850517, 1519.0197950996478, 1522.273970715093, 1525.527968696852, 1528.781789044925, 1532.0354317593121, 1535.288896840013, 1538.542184287028, 1541.7952941003568, 1545.0482262799999, 1548.300980825957, 1551.553557738228, 1554.8059570168132, 1558.058178661712, 1561.3102226729247, 1564.562089050452, 1567.813777794293, 1571.065288904448, 1574.3166223809171, 1577.5677782237, 1580.818756432797, 1584.0695570082078, 1587.320179949933, 1590.5706252579719, 1593.820892932325, 1597.070982972992, 1600.320895379973, 1603.570630153268, 1606.8201872928769, 1610.0695667987998, 1613.3187686710369, 1616.567792909588, 1619.816639514453, 1623.065308485632, 1626.313799823125, 1629.5621135269319, 1632.810249597053, 1636.058208033488, 1639.305988836237, 1642.5535920053, 1645.8010175406769, 1649.048265442368, 1652.295335710373, 1655.542228344692, 1658.788943345325, 1662.035480712272, 1665.2818404455331, 1668.528022545108, 1671.7740270109969, 1675.0198538431998, 1678.2655030417168, 1681.510974606548, 1684.756268537693, 1688.001384835152, 1691.246323498925, 1694.491084529012, 1697.7356679254128, 1700.980073688128, 1704.2243018171569, 1707.4683523125, 1710.712225174157, 1713.955920402128, 1717.199437996413, 1720.442777957012, 1723.685940283925, 1726.9289249771518, 1730.171732036693, 1733.4143614625482, 1736.656813254717, 1739.8990874132, 1743.1411839379969, 1746.3831028291079, 1749.624844086533, 1752.866407710272, 1756.1077937003251, 1759.349002056692, 1762.590032779373, 1765.830885868368, 1769.0715613236769, 1772.3120591453, 1775.552379333237, 1778.7925218874882, 1782.032486808053, 1785.272274094932, 1788.5118837481248, 1791.751315767632, 1794.990570153453, 1798.229646905588, 1801.468546024037, 1804.7072675088, 1807.945811359877, 1811.1841775772677, 1814.4223661609728, 1817.660377110992, 1820.898210427325, 1824.135866109972, 1827.373344158933, 1830.610644574208, 1833.8477673557968, 1837.0847125036998, 1840.3214800179169, 1843.5580698984481, 1846.7944821452932, 1850.030716758452, 1853.2667737379247, 1856.502653083712, 1859.738354795813, 1862.973878874228, 1866.2092253189571, 1869.44439413, 1872.679385307357, 1875.9141988510278, 1879.148834761013, 1882.383293037312, 1885.617573679925, 1888.851676688852, 1892.085602064093, 1895.319349805648, 1898.5529199135167, 1901.7863123876998, 1905.019527228197, 1908.252564435008, 1911.4854240081331, 1914.718105947572, 1917.9506102533248, 1921.182936925392, 1924.4150859637728, 1927.6470573684678, 1930.878851139477, 1934.1104672768001, 1937.341905780437, 1940.573166650388, 1943.804249886653, 1947.0351554892318, 1950.265883458125, 1953.496433793332, 1956.7268064948528, 1959.957001562688, 1963.187018996837, 1966.4168587973, 1969.646520964077, 1972.8760054971679, 1976.105312396573, 1979.3344416622917, 1982.563393294325, 1985.792167292672, 1989.020763657333, 1992.2491823883079, 1995.477423485597, 1998.7054869492, 2001.9333727791168, 2005.1610809753479, 2008.388611537893, 2011.615964466752, 2014.843139761925, 2018.070137423412, 2021.296957451213, 2024.523599845328, 2027.750064605757, 2030.9763517325, 2034.202461225557, 2037.4283930849278, 2040.6541473106129, 2043.879723902612, 2047.1051228609247, 2050.330344185552, 2053.5553878764927, 2056.7802539337476, 2060.004942357317, 2063.2294531472, 2066.453786303397, 2069.677941825908, 2072.901919714733, 2076.125719969872, 2079.349342591325, 2082.5727875790917, 2085.796054933173, 2089.019144653568, 2092.2420567402764, 2095.4647911933, 2098.687348012637, 2101.909727198288, 2105.131928750253, 2108.3539526685317, 2111.575798953125, 2114.797467604032, 2118.018958621253, 2121.240272004788, 2124.4614077546366, 2127.6823658708, 2130.903146353277, 2134.123749202068, 2137.344174417173, 2140.5644219985916, 2143.7844919463246, 2147.004384260372, 2150.224098940733, 2153.443635987408, 2156.662995400397, 2159.8821771797, 2163.101181325317, 2166.3200078372483, 2169.538656715493, 2172.757127960052, 2175.975421570925, 2179.193537548112, 2182.4114758916126, 2185.6292366014277, 2188.8468196775566, 2192.0642251199997, 2195.281452928757, 2198.498503103828, 2201.715375645213, 2204.932070552912, 2208.148587826925, 2211.364927467252, 2214.581089473893, 2217.797073846848, 2221.012880586117, 2224.2285096916994, 2227.4439611635967, 2230.6592350018077, 2233.874331206333, 2237.089249777172, 2240.3039907143248, 2243.5185540177918, 2246.732939687573, 2249.947147723668, 2253.161178126077, 2256.3750308948, 2259.588706029837, 2262.802203531188, 2266.015523398853, 2269.2286656328315, 2272.4416302331247, 2275.6544171997316, 2278.8670265326527, 2282.0794582318877, 2285.291712297437, 2288.5037887293, 2291.7156875274773, 2294.927408691968, 2298.1389522227732, 2301.350318119892, 2304.5615063833247, 2307.772517013072, 2310.983350009133, 2314.1940053715075, 2317.4044831001966, 2320.6147831952, 2323.824905656517, 2327.0348504841477, 2330.2446176780927, 2333.454207238352, 2336.663619164925, 2339.872853457812, 2343.081910117013, 2346.290789142528, 2349.499490534357, 2352.7080142925, 2355.916360416957, 2359.124528907728, 2362.332519764813, 2365.540332988212, 2368.747968577925, 2371.955426533952, 2375.162706856293, 2378.369809544948, 2381.576734599917, 2384.7834820212, 2387.990051808797, 2391.1964439627077, 2394.402658482933, 2397.608695369472, 2400.814554622325, 2404.0202362414916, 2407.225740226973, 2410.431066578768, 2413.636215296877, 2416.8411863813, 2420.045979832037, 2423.250595649088, 2426.455033832453, 2429.659294382132, 2432.863377298125, 2436.0672825804318, 2439.271010229053, 2442.474560243988, 2445.677932625237, 2448.8811273727997, 2452.084144486677, 2455.286983966868, 2458.489645813373, 2461.692130026192, 2464.894436605325, 2468.096565550772, 2471.2985168625332, 2474.500290540608, 2477.7018865849973, 2480.9033049956997, 2484.104545772717, 2487.305608916048, 2490.5064944256924, 2493.7072023016517, 2496.907732543925, 2500.1080851525116, 2503.3082601274127, 2506.508257468628, 2509.708077176157, 2512.90771925, 2516.107183690157, 2519.306470496628, 2522.5055796694132, 2525.704511208512, 2528.903265113925, 2532.101841385652, 2535.3002400236924, 2538.4984610280476, 2541.6965043987166, 2544.8943701357, 2548.0920582389967]
  in  "Stop":bool
  # "Fix multiplexer glitch\nsend notification button"
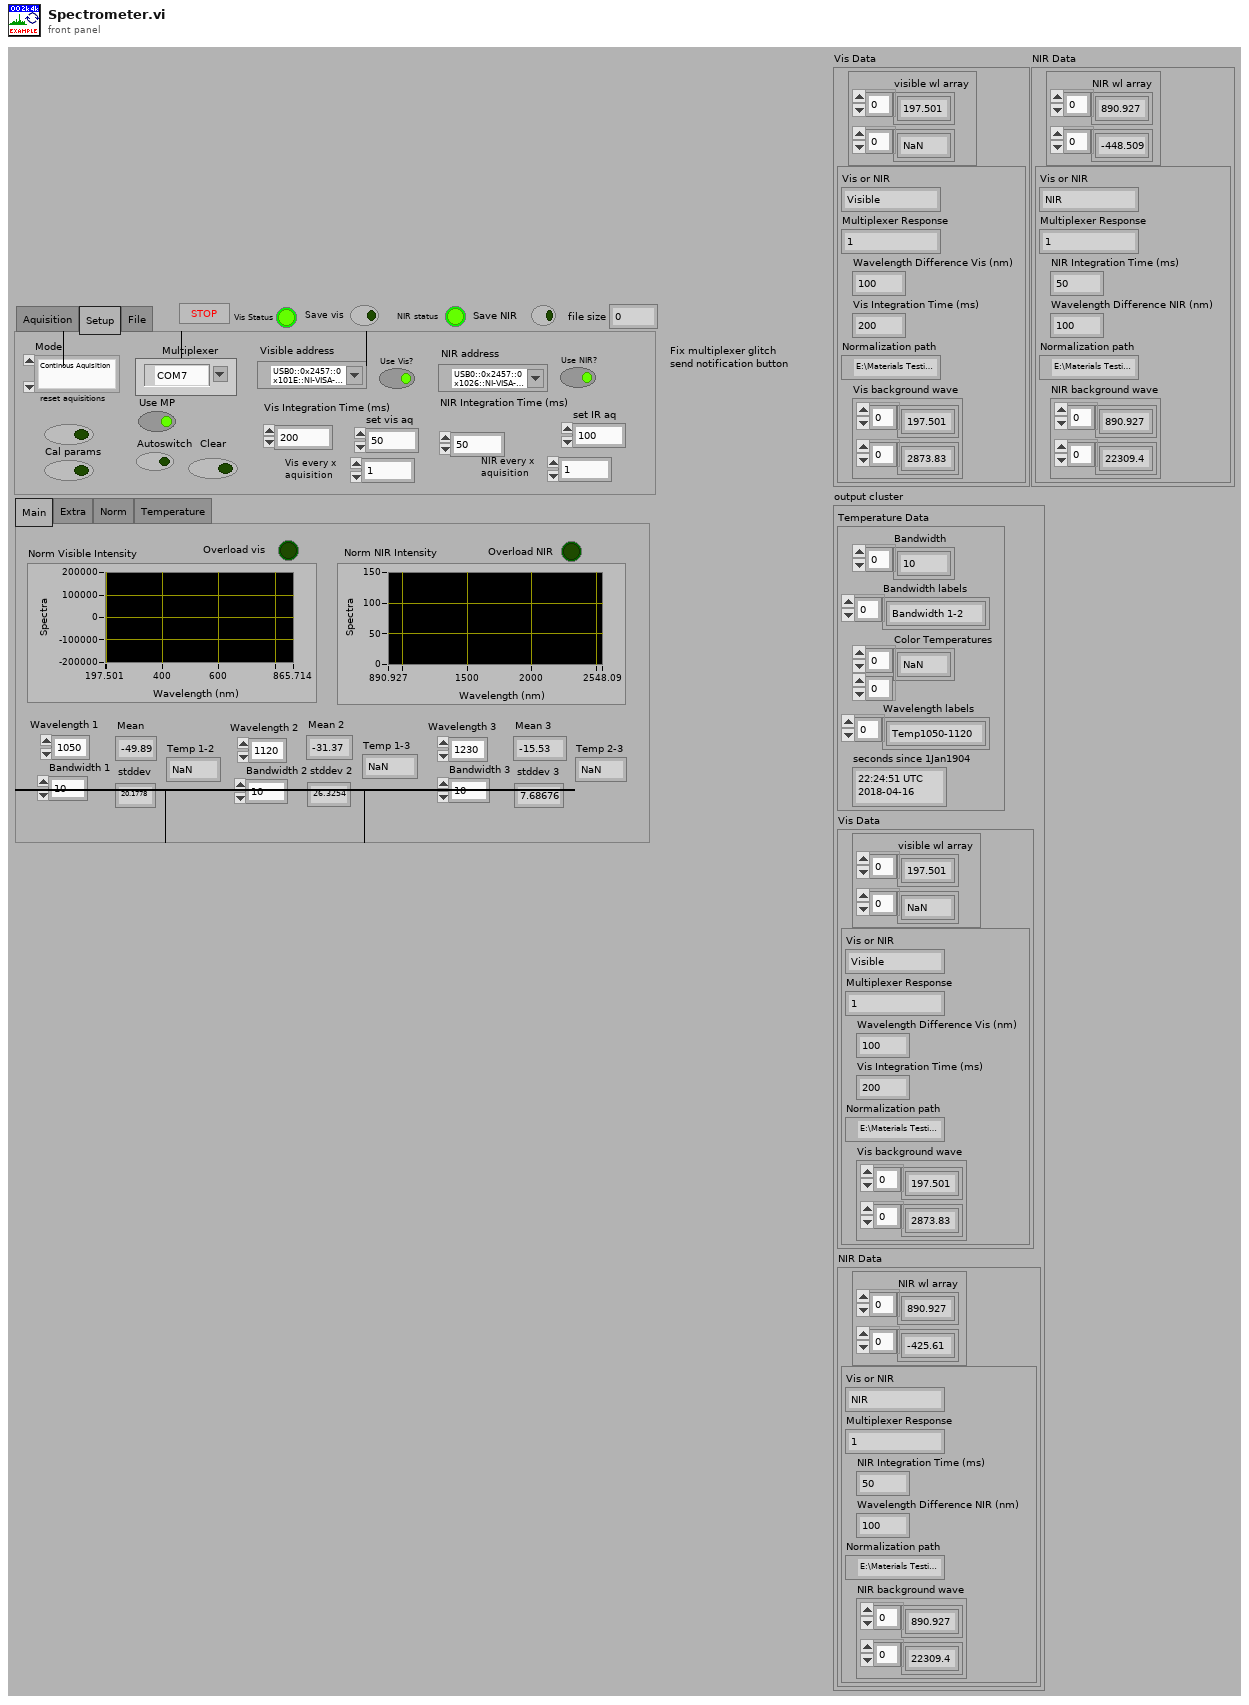
[diagram p1: front panel]
types:
  T1 = cluster{"Temperature Data":cluster{"Bandwidth":i32[], "Bandwidth labels":string[], "Color Temperatures":dbl[][], "Wavelength labels":string[], "seconds since 1Jan1904":timestamp}, "Vis Data":cluster{cluster{"visible wl array":dbl[], dbl[]}, cluster{"Vis or NIR":string, "Multiplexer Response":string, "Wavelength Difference Vis (nm)":dbl, "Vis Integration Time (ms)":u32, "Normalization path":path, "Vis background wave":cluster{dbl[], dbl[]}}}, "NIR Data":cluster{cluster{"NIR wl array":dbl[], dbl[]}, cluster{"Vis or NIR":string, "Multiplexer Response":string, "NIR Integration Time (ms)":u32, "Wavelength Difference NIR (nm) ":dbl, "Normalization path":path, "NIR background wave":cluster{dbl[], dbl[]}}}}
  T2 = cluster{cluster{"NIR wl array":dbl[], dbl[]}, cluster{"Vis or NIR":string, "Multiplexer Response":string, "NIR Integration Time (ms)":u32, "Wavelength Difference NIR (nm) ":dbl, "Normalization path":path, "NIR background wave":cluster{dbl[], dbl[]}}}
  T3 = cluster{cluster{"visible wl array":dbl[], dbl[]}, cluster{"Vis or NIR":string, "Multiplexer Response":string, "Wavelength Difference Vis (nm)":dbl, "Vis Integration Time (ms)":u32, "Normalization path":path, "Vis background wave":cluster{dbl[], dbl[]}}}
  T4 = enum16{"Move position", "Get Status", "Get Program"}
  T5 = enum16{"Continous Aquisition", "Single Aquisition", "Cont switch"}
  T6 = cluster{"Bandwidth":i32[], "Bandwidth labels":string[], "Color Temperatures":dbl[][], "Wavelength labels":string[], "seconds since 1Jan1904":timestamp}
  T7 = cluster{"baud rate":u32, "data bits":u16, "parity":enum16{"None", "Odd", "Even", "Mark", "Space"}, "stop bits":u16, "flow control":u16}
  T8 = cluster{"NIR wl array":dbl[], "Spectrum by Pixel Number":dbl[]}
  T9 = cluster{"Vis or NIR":string, "Multiplexer Response":string, "NIR Integration Time (ms)":u32, "Wavelength Difference NIR (nm) ":dbl, "Normalization path":path, "NIR background wave":cluster{dbl[], dbl[]}}
  T10 = cluster{"visible wl array":dbl[], "Spectrum by Pixel Number":dbl[]}
  T11 = cluster{"Vis or NIR":string, "Multiplexer Response":string, "Wavelength Difference Vis (nm)":dbl, "Vis Integration Time (ms)":u32, "Normalization path":path, "Vis background wave":cluster{dbl[], dbl[]}}
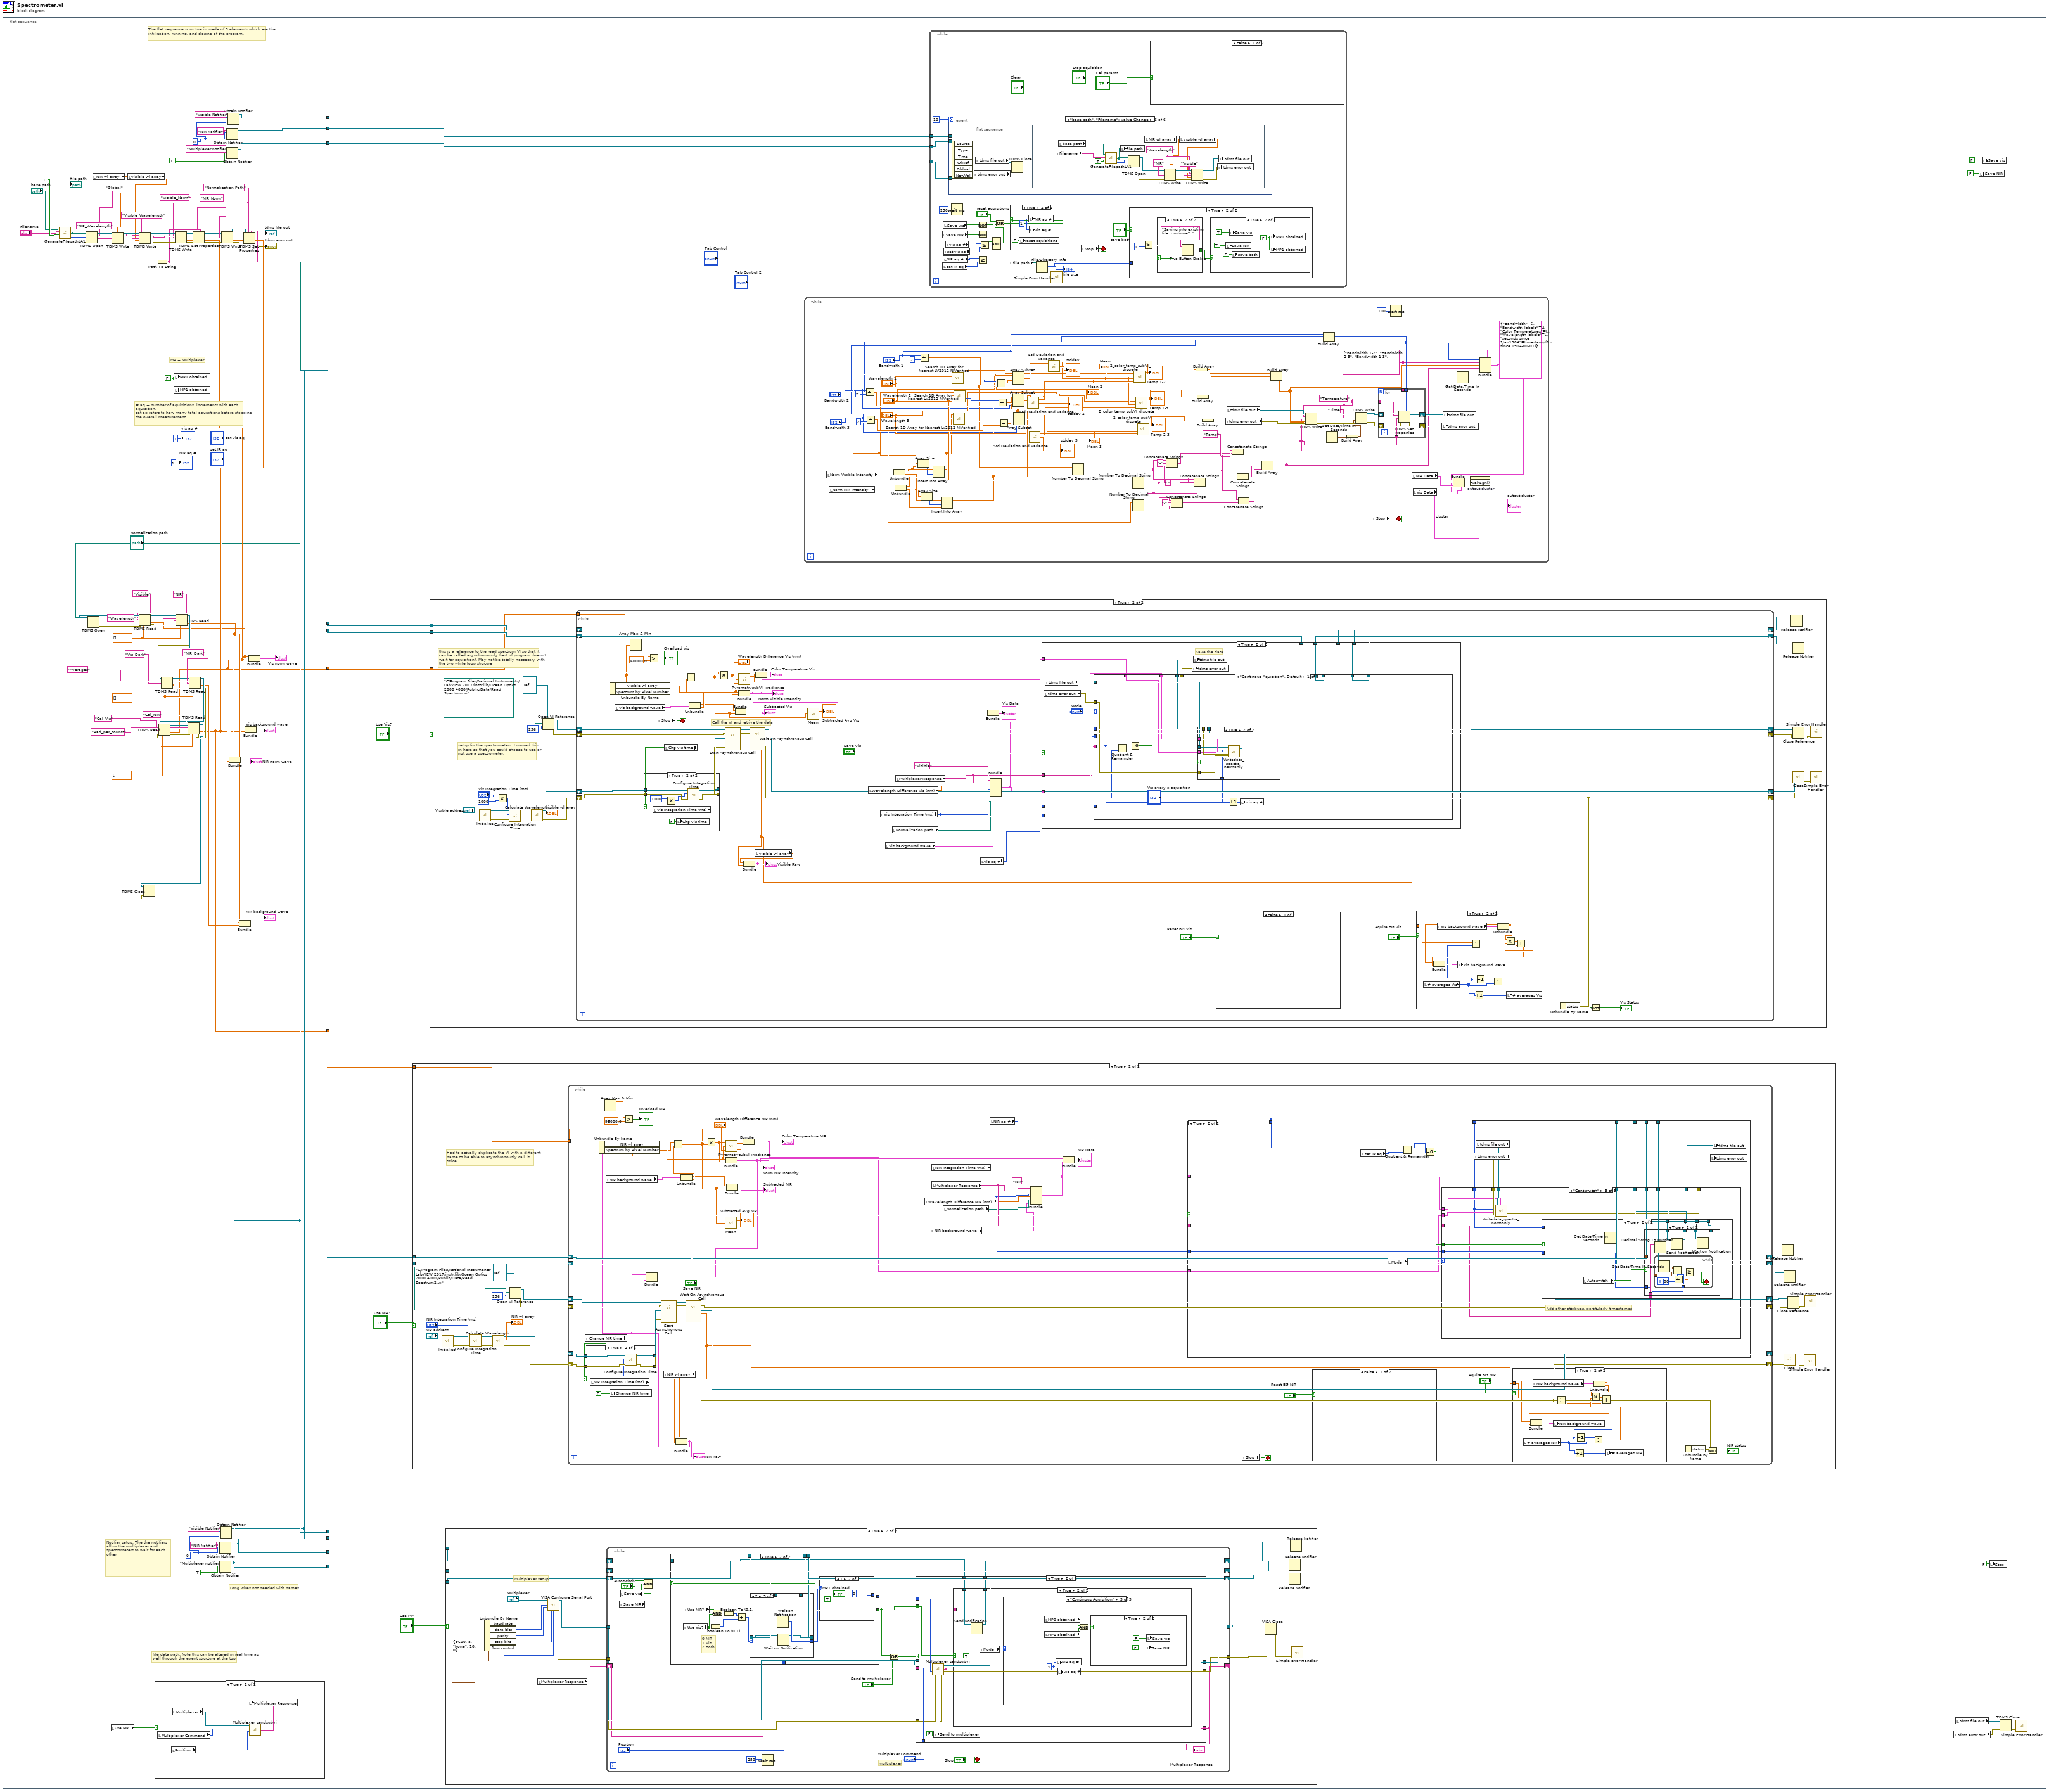
[diagram p0: block diagram]
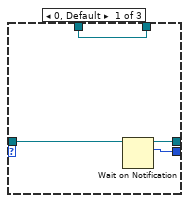
[diagram p5: hidden frame]
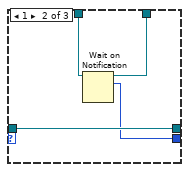
[diagram p6: hidden frame]
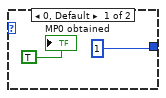
[diagram p7: hidden frame]
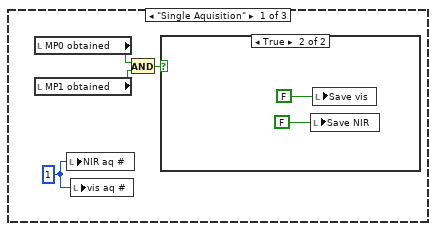
[diagram p10: hidden frame]
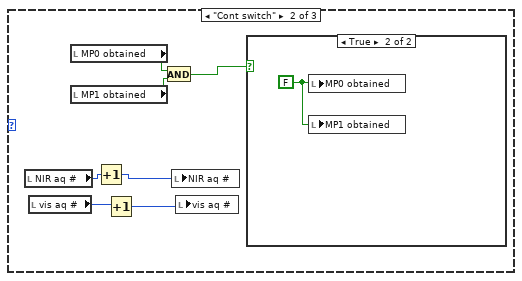
[diagram p12: hidden frame]
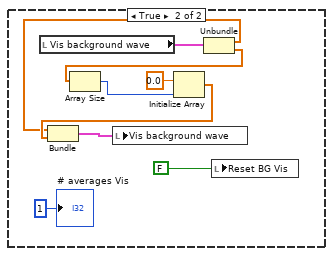
[diagram p17: hidden frame]
diagram:
  n1 = flat-sequence {
    tunnel: [w91] -> w12
    tunnel: [w90] -> w11
    tunnel: [w92] -> w10
    tunnel: [w92] -> w9
    tunnel: [w92] -> w8
    tunnel: [w91] -> w7
    tunnel: [w90] -> w6
    tunnel: [w42] -> w5
    tunnel: [w41] -> w4
    tunnel: [w48] -> w3
    tunnel: [w47] -> w2
    tunnel: [w46] -> w1
    tunnel: w12 -> [w124]
    tunnel: w11 -> [w119]
    tunnel: w10 -> [w120]
    tunnel: w9 -> [w123]
    tunnel: w8 -> [w118]
    tunnel: w7 -> [w121]
    tunnel: w6 -> [w122]
    tunnel: w5 -> [w114]
    tunnel: w4 -> [w113]
    tunnel: w3 -> [w112]
    tunnel: w2 -> [w111]
    tunnel: w1 -> [w110]
    frame #0 {
      w22 = "Normalization Path" ("group name in (Untitled)")
      w52 = 0
      w64 = dbl[] []
      w65 = dbl[] []
      w66 = dbl[] []
      w87 = FALSE ("save both")
      w89 = 0
      # "Long wires not needed with names"
      # "Notifier setup. The the notifiers allow the multiplexer and spectrometers to wait for each other"
      # "file data path. Note this can be altered in real time as well through the event structure at the top"
      # "# aq = number of aquisitions. increments with each aquisition.\nset aq refers to how many total aquisitions before stopping the overall measurement."
      # "MP = Multiplexer"
      # "The flat sequence scructure is made of 3 elements which are the intilization, running, and closing of the program."
      n2 = call "GenerateFilepathLA1.vi"("Auto Date folder"=TRUE, "Filename"="Filename", "base path"="base path") -> ("Numeric"=w14:i32, "file path"=w13:path)  [unwired: 1 in, 1 out]
      "file path" <- w13
      n3 = TDMS Open(10:w14, 11:w13) -> (0:w97:errorcluster, 3:w98:refnum<k34>)  [unwired: 5 in]
      n4 = TDMS Open(11:"Normalization path") -> (0:w83:errorcluster, 3:w84:refnum<k34>)  [unwired: 6 in]
      n5 = local read "NIR wl array"() -> (w99:dbl[])
      n6 = local read "Use MP"() -> (w45:bool)
      n7 = TDMS Write(0:w98, 5:"Global" ("group name in (Untitled)"), 7:"NIR_Wavelength" ("group name in (Untitled)"), 9:w99, 11:w97) -> (4:w102:refnum<k34>, 6:w38:string, 15:w103:errorcluster)  [unwired: 1 in, 1 out]
      n8 = local read "visible wl array"() -> (w96:dbl[])
      n9 = TDMS Write(0:w102, 5:w38, 7:"Visible_Wavelength" ("group name in (Untitled)"), 9:w96, 11:w103) -> (4:w44:refnum<k34>, 6:w39:string, 15:w43:errorcluster)  [unwired: 1 in, 1 out]
      n10 = TDMS Read(0:w84, 5:"Wavelength" ("group name in"), 7:"Visible", 11:w83, 12:w66) -> (4:w79:refnum<k34>, 6:w78:string, 10:w19:dbl[], 15:w77:errorcluster)  [unwired: 3 in, 2 out]
      n11 = case shown="True" w45 {
        frame False {
        }
        frame True {
          n12 = local read "Multiplexer Command"() -> (w108:T4)
          n13 = local read "Position"() -> (w107:i32)
          n14 = local read "Multiplexer"() -> (w109:refnum<visa-resource-name>)
          n15 = call "Multiplexer_sendsubvi.vi"("Position"=w107, "Enum"=w108, "VISA resource name"=w109) -> ("Response"=w106:string)  [unwired: 1 in, 2 out]
          n16 = local write "Multiplexer Response"(w106) -> ()
        }
      }
      n17 = Path To String(path="Normalization path") -> (string=w25:string)
      n18 = local write "MP0 obtained"(w87) -> ()
      n19 = local write "MP1 obtained"(w87) -> ()
      n20 = TDMS Read(0:w79, 5:w78, 7:"NIR", 11:w77, 12:w66) -> (4:w61:refnum<k34>, 10:w55:dbl[], 15:w60:errorcluster)  [unwired: 3 in, 3 out]
      n21 = TDMS Read(0:w61, 5:"Averages" ("group name in"), 7:"Vis_Dark", 11:w60, 12:w65) -> (4:w63:refnum<k34>, 6:w76:string, 10:w18:dbl[], 15:w75:errorcluster)  [unwired: 3 in, 2 out]
      n22 = TDMS Read(0:w63, 5:w76, 7:"NIR_Dark", 11:w75, 12:w65) -> (4:w59:refnum<k34>, 10:w54:dbl[], 15:w58:errorcluster)  [unwired: 3 in, 3 out]
      n23 = TDMS Read(0:w59, 5:"Rad_per_counts" ("group name in"), 7:"Cal_Vis", 11:w58, 12:w64) -> (4:w74:refnum<k34>, 6:w73:string, 10:w42:dbl[], 15:w62:errorcluster)  [unwired: 3 in, 2 out]
      n24 = TDMS Write(0:w44, 5:w39, 7:"Visible_Norm" ("group name in (Untitled)"), 9:w42, 11:w43) -> (4:w31:refnum<k34>, 6:w32:string, 8:w33:string, 15:w34:errorcluster)  [unwired: 1 in]
      n25 = TDMS Read(0:w74, 5:w73, 7:"Cal_NIR", 11:w62, 12:w64) -> (4:w57:refnum<k34>, 10:w41:dbl[], 15:w56:errorcluster)  [unwired: 3 in, 3 out]
      n26 = TDMS Close(8:w56, 11:w57) -> ()  [unwired: 2 out]
      n27 = TDMS Set Properties(5:w25, 7:w22, 8:w34, 9:w33, 10:w32, 11:w31) -> (0:w29:errorcluster, 2:w28:string, 3:w30:refnum<k34>)  [unwired: 1 out]
      n28 = Obtain Notifier(name (unnamed)="NIR Notifier", notification data type=w89) -> (notifier out=w91:refnum<notifier>)  [unwired: 2 in, 2 out]
      n29 = Obtain Notifier(name (unnamed)="Multiplexer notifier", notification data type=TRUE) -> (notifier out=w92:refnum<notifier>)  [unwired: 2 in, 2 out]
      n30 = Obtain Notifier(name (unnamed)="Visible Notifier", notification data type=w89) -> (notifier out=w90:refnum<notifier>)  [unwired: 2 in, 2 out]
      n31 = TDMS Write(0:w30, 5:w28, 7:"NIR_Norm" ("group name in (Untitled)"), 9:w41, 11:w29) -> (4:w26:refnum<k34>, 6:w24:string, 8:w23:string, 15:w27:errorcluster)  [unwired: 1 in]
      n32 = Obtain Notifier(name (unnamed)="NIR Notifier", notification data type=w52) -> (notifier out=w47:refnum<notifier>)  [unwired: 2 in, 2 out]
      n33 = Obtain Notifier(name (unnamed)="Multiplexer notifier", notification data type=TRUE) -> (notifier out=w46:refnum<notifier>)  [unwired: 2 in, 2 out]
      n34 = Obtain Notifier(name (unnamed)="Visible Notifier", notification data type=w52) -> (notifier out=w48:refnum<notifier>)  [unwired: 2 in, 2 out]
      n35 = Bundle(w55, w41) -> (→"NIR norm wave":cluster{dbl[], dbl[]})  [unwired: 1 out]
      n36 = Bundle(w55, w54) -> ()  [unwired: 2 out]
      n37 = TDMS Set Properties(5:w25, 7:w22, 8:w27, 9:w23, 10:w24, 11:w26) -> (0:→"tdms error out":errorcluster, 3:→"tdms file out":refnum<k34>)  [unwired: 2 out]
      n38 = Bundle(w19, w18) -> ()  [unwired: 2 out]
      n39 = Bundle(w19, w42) -> (→"Vis norm wave":cluster{dbl[], dbl[]})  [unwired: 1 out]
      "NIR aq #" <- 1 ("# NIR aq")
      "vis aq #" <- 1 ("Numeric")
    }
    frame #1 {
      n40 = case shown="True" "Use NIR?" {
        tunnel: w124 -> [_ w600]
        tunnel: w123 -> [_ w599]
        tunnel: w113 -> [_ w578]
        frame False {
        }
        frame True {
          # "Had to actually duplicate the VI with a different name to be able to asynchronously call is twice...."
          n41 = call <instrlib>:"Initialize.vi"("VISA resource name"="NIR address") -> ("error out"=w594:errorcluster, "VISA resource name out"=w596:refnum<visa-resource-name>)  [unwired: 2 in, 7 out]
          n42 = call <instrlib>:"Configure Integration Time.vi"("error in (no error)"=w594, "Integration Time (6000)"="NIR Integration Time (ms)", "VISA resource name"=w596) -> ("error out"=w593:errorcluster, "VISA resource name out"=w595:refnum<visa-resource-name>)  [unwired: 7 in]
          n43 = call <instrlib>:"Calculate Wavelength.vi"("error in (no error)"=w593, "VISA resource name"=w595) -> ("error out"=w585:errorcluster, "Wavelength (nm)"=→"NIR wl array":dbl[], "VISA resource name out"=w586:refnum<visa-resource-name>)  [unwired: 1 in, 6 out]
          n44 = Open VI Reference(type specifier VI Refnum (for type only)=refnum<vi> refnum, vi path=path "C:/Program Files/National Instruments/LabVIEW 2017/instr.lib/Ocean Optics 2000 4000/Public/Data/Read Spectrum2.vi", options=256) -> (vi reference=w588:refnum<vi>, error out=w587:errorcluster)  [unwired: 3 in]
          n45 = while {
            shift-right: [w648] -> w582
            shift-left: w588 -> [w651]
            shift-right: [w647] -> w581
            shift-left: w587 -> [w644]
            shift-right: [w638] -> w579
            shift-left: w585 -> [w641]
            shift-right: [w649] -> w580
            shift-left: w586 -> [w643]
            shift-right: [w637] -> w576
            shift-left: w600 -> [w632]
            shift-right: [w636] -> w577
            shift-left: w599 -> [w633]
            tunnel: w578 -> [w623]
            stop <- w646 stop-if-true
            n46 = local read "Change NIR time"() -> (w642:bool)
            n47 = case shown="True" w642 {
              tunnel: [w676 w679] -> w640
              tunnel: w643 -> [w676 w682]
              tunnel: [w675 w680] -> w639
              tunnel: w641 -> [w675 w681]
              frame False {
              }
              frame True {
                n48 = local read "NIR Integration Time (ms)"() -> (w677:u32)
                n49 = local write "Change NIR time"(FALSE ("Chg vis time")) -> ()
                n50 = call <instrlib>:"Configure Integration Time.vi"("error in (no error)"=w681, "Integration Time (6000)"=w677, "VISA resource name"=w682) -> ("error out"=w680:errorcluster, "VISA resource name out"=w679:refnum<visa-resource-name>)  [unwired: 7 in]
              }
            }
            n51 = local read "NIR background wave"() -> (w621:cluster{dbl[], dbl[]})
            n52 = call-by-ref "Start Asynchronous Call"(reference=w651, error in=w644, 8:"error in (no error)"=w639, "VISA resource name"=w640) -> (reference out=w653:refnum<vi>, error out=w650:errorcluster)  [unwired: 6 in, 4 out]
            n53 = local read "NIR wl array"() -> (w652:dbl[])
            n54 = Unbundle(w621) -> (w613:dbl[], w620:dbl[])
            n55 = call-by-ref "Wait On Asynchronous Call"(reference=w653, error in=w650) -> (reference out=w648:refnum<vi>, error out=w647:errorcluster, 0:"error out"=w638:errorcluster, "Spectrum by Pixel Number"=w617:dbl[], "VISA resource name out"=w649:refnum<visa-resource-name>)  [unwired: 8 in, 1 out]
            n56 = Bundle("NIR wl array"=w652, "Spectrum by Pixel Number"=w617) -> (w622:T8)  [unwired: 1 out]
            "NIR Raw" <- w622
            n57 = Unbundle By Name(w622) -> ("NIR wl array"=w625:dbl[], "Spectrum by Pixel Number"=w615:dbl[])
            n58 = Array Max & Min(array=w615) -> (max value=w628:dbl)  [unwired: 3 out]
            n59 = Greater?(x=w628, y=95000.0) -> (0:→"Overload NIR":bool)
            n60 = Subtract(x=w615, y=w620) -> (x-y=w612:dbl[])
            n61 = Multiply(x=w623, y=w612) -> (x*y=w624:dbl[])
            n62 = call-poly <vilib>:"Mean.vi"("X"=w612) -> ("mean"=→"Subtracted Avg NIR":dbl)  [unwired: 1 out]
            n63 = call "PyrometrysubVI_irradiance.vi"("Wavelength Difference (nm)"="Wavelength Difference NIR (nm)", "Wavelength in"=w625, "Data In"=w624) -> ("wl out"=w629:dbl[], "FT"=w630:dbl[])
            n64 = Bundle("NIR wl array"=w625, w624) -> (w607:cluster{"NIR wl array":dbl[], dbl[]})  [unwired: 1 out]
            "Norm NIR Intensity" <- w607
            n65 = Bundle(w613, w612) -> (→"Subtracted NIR":cluster{dbl[], dbl[]})  [unwired: 1 out]
            n66 = Bundle("wl out"=w629, "FT"=w630) -> (w601:cluster{"wl out":dbl[], "FT":dbl[]})  [unwired: 1 out]
            "Color Temperature NIR" <- w601
            n67 = Bundle(w622, w607, w601) -> ()  [unwired: 1 in, 1 out]
            n68 = local read "Wavelength Difference NIR (nm)"() -> (w605:dbl)
            n69 = local read "NIR background wave"() -> (w603:cluster{dbl[], dbl[]})
            n70 = local read "NIR Integration Time (ms)"() -> (w606:u32)
            n71 = local read "Multiplexer Response"() -> (w609:string)
            n72 = local read "Normalization path"() -> (w604:path)
            n73 = local read "NIR aq #"() -> (w608:i32)
            n74 = Bundle("Vis or NIR"="NIR", "Multiplexer Response"=w609, "NIR Integration Time (ms)"=w606, "Wavelength Difference NIR (nm)"=w605, "Normalization path"=w604, "NIR background wave"=w603) -> (w610:T9)  [unwired: 1 in]
            n75 = Bundle(w607, w610) -> (→"NIR Data":T2)  [unwired: 1 in]
            n76 = case shown="True" "Save NIR" {
              tunnel: w632 -> [w684 w702]
              tunnel: w633 -> [w683 w701]
              tunnel: [w684 w700] -> w637
              tunnel: [w683 w699] -> w636
              tunnel: w601 -> [_ w690]
              tunnel: w610 -> [_ w689]
              tunnel: w606 -> [_ w688]
              tunnel: w609 -> [_ w687]
              tunnel: w608 -> [_ w686]
              tunnel: w608 -> [_ w685]
              frame False {
              }
              frame True {
                n77 = local read "set IR aq"() -> (w693:i32)
                n78 = local read "Mode"() -> (w698:T5)
                n79 = Quotient & Remainder(x=w686, y=w693) -> (x-y*floor(x/y)=w692:i32)  [unwired: 1 out]
                n80 = Equal To 0?(x=w692) -> (x = 0?=w691:bool)
                n81 = local read "tdms error out"() -> (w697:errorcluster)
                n82 = local read "tdms file out"() -> (w696:refnum<k34>)
                n83 = case shown="\"Cont switch\"" w698 {
                  tunnel: w691 -> [_ w738 w782]
                  tunnel: w702 -> [w715 w737 w781]
                  tunnel: w701 -> [w714 w736 w780]
                  tunnel: [w715 w735 w779] -> w700
                  tunnel: [w714 w734 w778] -> w699
                  tunnel: w688 -> [_ w733 w777]
                  tunnel: w685 -> [w703 w725 w769]
                  tunnel: w687 -> [_ w732 w776]
                  tunnel: w690 -> [w708 w731 w770]
                  tunnel: w689 -> [w709 w726 w771]
                  tunnel: w697 -> [w712 w730 w775]
                  tunnel: w696 -> [w713 w729 w774]
                  tunnel: [w710 w728 w773] -> w695
                  tunnel: [w711 w727 w772] -> w694
                  frame "Continous Aquisition", Default {
                    n84 = Quotient & Remainder(x=w703, y="NIR every x aquisition") -> (x-y*floor(x/y)=w706:i32)  [unwired: 1 out]
                    n85 = Increment(x=w703) -> (x+1=w704:i32)
                    n86 = Equal To 0?(x=w706) -> (x = 0?=w705:bool)
                    n87 = local write "NIR aq #"(w704) -> ()
                    n88 = case shown="True" w705 {
                      tunnel: w713 -> [w717 w724]
                      tunnel: w712 -> [w716 w723]
                      tunnel: [w717 w722] -> w711
                      tunnel: [w716 w721] -> w710
                      tunnel: w709 -> [_ w720]
                      tunnel: w708 -> [_ w719]
                      tunnel: w703 -> [_ w718]
                      frame False {
                      }
                      frame True {
                        n89 = call "Writedata_spectra_normonly.vi"("tdms file in"=w724, "Aquisition number"=w718, "Norm Visible Intensity"=w719, "tdms error in"=w723, "Params"=w720) -> ("tdms file out"=w722:refnum<k34>, "tdms error out"=w721:errorcluster)
                      }
                    }
                  }
                  frame "Single Aquisition" {
                    # "Add other attribues, partitularly timestamps"
                    n90 = call "Writedata_spectra_normonly.vi"("tdms file in"=w729, "Aquisition number"=w725, "Norm Visible Intensity"=w731, "tdms error in"=w730, "Params"=w726) -> ("tdms file out"=w727:refnum<k34>, "tdms error out"=w728:errorcluster)
                    n91 = case shown="True" w738 {
                      tunnel: w737 -> [w742 w748]
                      tunnel: w736 -> [w741 w746]
                      tunnel: w732 -> [_ w749]
                      tunnel: [w742 w747] -> w735
                      tunnel: [w741 w745] -> w734
                      tunnel: w725 -> [w739 _]
                      tunnel: w733 -> [_ w743]
                      frame False {
                        n92 = Increment(x=w739) -> (x+1=w740:i32)
                        n93 = local write "NIR aq #"(w740) -> ()
                      }
                      frame True {
                        n94 = local read "Autoswitch"() -> (w750:bool)
                        n95 = Get Date/Time In Seconds() -> (seconds since 1Jan1904=w744:timestamp)
                        n96 = case shown="True" w750 {
                          tunnel: w749 -> [_ w761]
                          tunnel: w748 -> [w752 w759]
                          tunnel: [w752 w758] -> w747
                          tunnel: w746 -> [w751 w757]
                          tunnel: [w751 w756] -> w745
                          tunnel: w744 -> [_ w755]
                          tunnel: w743 -> [_ w754]
                          frame False {
                            n97 = local write "Save NIR"(FALSE ("Save Data")) -> ()
                          }
                          frame True {
                            n98 = while {
                              tunnel: w755 -> [w767]
                              tunnel: w754 -> [w764]
                              stop <- w765 stop-if-true
                              n99 = Get Date/Time In Seconds() -> (seconds since 1Jan1904=w768:timestamp)
                              n100 = Subtract(x=w768, y=w767) -> (x-y=w766:dbl)
                              n101 = Divide(x=w764, y=u32 1000) -> (x/y=w762:dbl)
                              n102 = Greater Or Equal?(x=w766, y=w762) -> (x >= y?=w765:bool)
                            }
                            n103 = Decimal String To Number(string=w761) -> (number=w760:i32)  [unwired: 2 in, 1 out]
                            n104 = Send Notification(notification=w760, notifier=w759) -> (notifier out=w758:refnum<notifier>)  [unwired: 1 in, 1 out]
                            n105 = Wait on Notification(notifier=w757) -> (notifier out=w756:refnum<notifier>)  [unwired: 3 in, 3 out]
                          }
                        }
                      }
                    }
                  }
                  frame "Cont switch" {
                    # "Add other attribues, partitularly timestamps"
                    n106 = call "Writedata_spectra_normonly.vi"("tdms file in"=w774, "Aquisition number"=w769, "Norm Visible Intensity"=w770, "tdms error in"=w775, "Params"=w771) -> ("tdms file out"=w772:refnum<k34>, "tdms error out"=w773:errorcluster)
                    n107 = case shown="True" w782 {
                      tunnel: w781 -> [w786 w792]
                      tunnel: w780 -> [w785 w790]
                      tunnel: w776 -> [_ w793]
                      tunnel: [w786 w791] -> w779
                      tunnel: [w785 w789] -> w778
                      tunnel: w769 -> [w783 _]
                      tunnel: w777 -> [_ w787]
                      frame False {
                        n108 = Increment(x=w783) -> (x+1=w784:i32)
                        n109 = local write "NIR aq #"(w784) -> ()
                      }
                      frame True {
                        n110 = local read "Autoswitch"() -> (w794:bool)
                        n111 = Get Date/Time In Seconds() -> (seconds since 1Jan1904=w788:timestamp)
                        n112 = case shown="True" w794 {
                          tunnel: w793 -> [_ w805]
                          tunnel: w792 -> [w796 w803]
                          tunnel: [w796 w802] -> w791
                          tunnel: w790 -> [w795 w801]
                          tunnel: [w795 w800] -> w789
                          tunnel: w788 -> [_ w799]
                          tunnel: w787 -> [_ w798]
                          frame False {
                            n113 = local write "Save NIR"(FALSE ("Save Data")) -> ()
                          }
                          frame True {
                            n114 = while {
                              tunnel: w799 -> [w811]
                              tunnel: w798 -> [w808]
                              stop <- w809 stop-if-true
                              n115 = Get Date/Time In Seconds() -> (seconds since 1Jan1904=w812:timestamp)
                              n116 = Subtract(x=w812, y=w811) -> (x-y=w810:dbl)
                              n117 = Divide(x=w808, y=u32 1000) -> (x/y=w806:dbl)
                              n118 = Greater Or Equal?(x=w810, y=w806) -> (x >= y?=w809:bool)
                            }
                            n119 = Decimal String To Number(string=w805) -> (number=w804:i32)  [unwired: 2 in, 1 out]
                            n120 = Send Notification(notification=w804, notifier=w803) -> (notifier out=w802:refnum<notifier>)  [unwired: 1 in, 1 out]
                            n121 = Wait on Notification(notifier=w801) -> (notifier out=w800:refnum<notifier>)  [unwired: 3 in, 3 out]
                          }
                        }
                      }
                    }
                  }
                }
                n122 = local write "tdms error out"(w695) -> ()
                n123 = local write "tdms file out"(w694) -> ()
              }
            }
            n124 = local read "Stop"() -> (w646:bool)
            n125 = case shown="False" "Reset BG NIR" {
              frame False {
              }
              frame True {
                n126 = local read "NIR background wave"() -> (w674:cluster{dbl[], dbl[]})
                n127 = Unbundle(w674) -> (w667:dbl[], w673:dbl[])
                n128 = Array Size(array=w673) -> (size(s)=w672:i32)
                n129 = Initialize Array(0.0 ("element"), w672) -> (w669:dbl[])
                n130 = Bundle(w667, w669) -> (w670:cluster{dbl[], dbl[]})  [unwired: 1 in]
                n131 = local write "NIR background wave"(w670) -> ()
                n132 = local write "Reset BG NIR"(FALSE ("Reset Background Vis")) -> ()
                "# averages NIR" <- 1 ("# averages")
              }
            }
            n133 = case shown="True" "Aquire BG NIR" {
              tunnel: w617 -> [_ w656]
              frame False {
              }
              frame True {
                n134 = local read "# averages NIR"() -> (w658:i32)
                n135 = local read "NIR background wave"() -> (w665:cluster{dbl[], dbl[]})
                n136 = Divide(x=w656, y=w658) -> (x/y=w655:dbl[])
                n137 = Increment(x=w658) -> (x+1=w657:i32)
                n138 = Decrement(x=w658) -> (x-1=w661:i32)
                n139 = Divide(x=w661, y=w658) -> (x/y=w660:dbl)
                n140 = Unbundle(w665) -> (w663:dbl[], w662:dbl[])
                n141 = Multiply(x=w662, y=w660) -> (x*y=w659:dbl[])
                n142 = Add(x=w659, y=w655) -> (x+y=w654:dbl[])
                n143 = Bundle(w663, w654) -> (w664:cluster{dbl[], dbl[]})  [unwired: 1 in]
                n144 = local write "NIR background wave"(w664) -> ()
                n145 = local write "# averages NIR"(w657) -> ()
              }
            }
            n146 = Unbundle By Name(w638) -> ("status"=w635:bool)
            n147 = Not(x=w635) -> (.not. x?=→"NIR status":bool)
          }
          n148 = Release Notifier(notifier=w577) -> ()  [unwired: 2 in, 3 out]
          n149 = Release Notifier(notifier=w576) -> ()  [unwired: 2 in, 3 out]
          n150 = call <instrlib>:"Close.vi"("error in (no error)"=w579, "VISA resource name"=w580) -> ("error out"=w583:errorcluster)  [unwired: 9 out]
          n151 = Close Reference(reference=w582, error in (no error)=w581) -> (error out=w584:errorcluster)
          n152 = call <vilib>:"Simple Error Handler.vi"("error in (no error)"=w583) -> ()  [unwired: 1 in, 8 out]
          n153 = call <vilib>:"Simple Error Handler.vi"("error in (no error)"=w584) -> ()  [unwired: 1 in, 8 out]
        }
      }
      n154 = case shown="True" "Use Vis?" {
        tunnel: w119 -> [_ w358]
        tunnel: w118 -> [_ w357]
        tunnel: w114 -> [_ w334]
        frame False {
        }
        frame True {
          # "this is a reference to the read spectrum VI so that it can be called asynchronously (rest of program doesn't wait for aquisition). May not be totally nessecary with the two while loop strucure"
          # "setup for the spectrometers. I moved this in here so that you could choose to use or not use a spectrometer."
          n155 = call <instrlib>:"Initialize.vi"("VISA resource name"="Visible address") -> ("error out"=w351:errorcluster, "VISA resource name out"=w352:refnum<visa-resource-name>)  [unwired: 2 in, 7 out]
          n156 = Multiply(x="Vis Integration Time (ms)", y=u32 1000) -> (x*y=w345:u32)
          n157 = call <instrlib>:"Configure Integration Time.vi"("error in (no error)"=w351, "Integration Time (6000)"=w345, "VISA resource name"=w352) -> ("error out"=w349:errorcluster, "VISA resource name out"=w350:refnum<visa-resource-name>)  [unwired: 7 in]
          n158 = call <instrlib>:"Calculate Wavelength.vi"("error in (no error)"=w349, "VISA resource name"=w350) -> ("error out"=w341:errorcluster, "Wavelength (nm)"=→"visible wl array":dbl[], "VISA resource name out"=w342:refnum<visa-resource-name>)  [unwired: 1 in, 6 out]
          n159 = Open VI Reference(type specifier VI Refnum (for type only)=refnum<vi> refnum, vi path=path "C:/Program Files/National Instruments/LabVIEW 2017/instr.lib/Ocean Optics 2000 4000/Public/Data/Read Spectrum.vi", options=256) -> (vi reference=w344:refnum<vi>, error out=w343:errorcluster)  [unwired: 3 in]
          n160 = while {
            shift-right: [w407] -> w336
            shift-left: w344 -> [w409]
            shift-right: [w396] -> w337
            shift-left: w341 -> [w399]
            shift-right: [w406] -> w335
            shift-left: w343 -> [w402]
            shift-right: [w408] -> w338
            shift-left: w342 -> [w400]
            shift-right: [w395] -> w332
            shift-left: w358 -> [w391]
            shift-right: [w394] -> w333
            shift-left: w357 -> [w390]
            tunnel: w334 -> [w389]
            stop <- w405 stop-if-true
            # "Call the VI and retrive the data"
            n161 = local read "Vis background wave"() -> (w377:cluster{dbl[], dbl[]})
            n162 = local read "Stop"() -> (w405:bool)
            n163 = local read "Chg vis time"() -> (w401:bool)
            n164 = case shown="True" w401 {
              tunnel: [w434 w439] -> w398
              tunnel: w400 -> [w434 w442]
              tunnel: [w433 w440] -> w397
              tunnel: w399 -> [w433 w441]
              frame False {
              }
              frame True {
                n165 = local read "Vis Integration Time (ms)"() -> (w437:u32)
                n166 = Multiply(x=u32 1000, y=w437) -> (x*y=w435:u32)
                n167 = local write "Chg vis time"(FALSE ("Chg vis time")) -> ()
                n168 = call <instrlib>:"Configure Integration Time.vi"("error in (no error)"=w441, "Integration Time (6000)"=w435, "VISA resource name"=w442) -> ("error out"=w440:errorcluster, "VISA resource name out"=w439:refnum<visa-resource-name>)  [unwired: 7 in]
              }
            }
            n169 = Unbundle(w377) -> (w371:dbl[], w376:dbl[])
            n170 = call-by-ref "Start Asynchronous Call"(reference=w409, error in=w402, 8:"error in (no error)"=w397, "VISA resource name"=w398) -> (reference out=w411:refnum<vi>, error out=w410:errorcluster)  [unwired: 6 in, 4 out]
            n171 = call-by-ref "Wait On Asynchronous Call"(reference=w411, error in=w410) -> (reference out=w407:refnum<vi>, error out=w406:errorcluster, 0:"error out"=w396:errorcluster, "Spectrum by Pixel Number"=w373:dbl[], "VISA resource name out"=w408:refnum<visa-resource-name>)  [unwired: 8 in, 1 out]
            n172 = local read "visible wl array"() -> (w404:dbl[])
            n173 = Bundle("visible wl array"=w404, "Spectrum by Pixel Number"=w373) -> (w379:T10)  [unwired: 1 out]
            "Visible Raw" <- w379
            n174 = Unbundle By Name(w379) -> ("visible wl array"=w381:dbl[], "Spectrum by Pixel Number"=w385:dbl[])
            n175 = Array Max & Min(array=w385) -> (max value=w384:dbl)  [unwired: 3 out]
            n176 = Greater?(x=w384, y=60000.0) -> (0:→"Overload vis":bool)
            n177 = Subtract(x=w385, y=w376) -> (x-y=w369:dbl[])
            n178 = Multiply(x=w389, y=w369) -> (x*y=w380:dbl[])
            n179 = Bundle(w371, w369) -> (→"Subtracted Vis":cluster{dbl[], dbl[]})  [unwired: 1 out]
            n180 = call "PyrometrysubVI_irradiance.vi"("Wavelength Difference (nm)"="Wavelength Difference Vis (nm)", "Wavelength in"=w381, "Data In"=w380) -> ("wl out"=w386:dbl[], "FT"=w387:dbl[])
            n181 = Bundle("visible wl array"=w381, w380) -> (w363:cluster{"visible wl array":dbl[], dbl[]})  [unwired: 1 out]
            "Norm Visible Intensity" <- w363
            n182 = Bundle("wl out"=w386, "FT"=w387) -> (→"Color Temperature Vis":cluster{"wl out":dbl[], "FT":dbl[]})  [unwired: 1 out]
            n183 = call-poly <vilib>:"Mean.vi"("X"=w369) -> ("mean"=→"Subtracted Avg Vis":dbl)  [unwired: 1 out]
            n184 = local read "Wavelength Difference Vis (nm)"() -> (w365:dbl)
            n185 = local read "Vis Integration Time (ms)"() -> (w367:u32)
            n186 = local read "Vis background wave"() -> (w359:cluster{dbl[], dbl[]})
            n187 = local read "Normalization path"() -> (w364:path)
            n188 = local read "Multiplexer Response"() -> (w366:string)
            n189 = local read "vis aq #"() -> (w361:i32)
            n190 = Bundle("Vis or NIR"="Visible", "Multiplexer Response"=w366, "Wavelength Difference Vis (nm)"=w365, "Vis Integration Time (ms)"=w367, "Normalization path"=w364, "Vis background wave"=w359) -> (w362:T11)  [unwired: 1 in]
            n191 = Bundle(w363, w362) -> (→"Vis Data":T3)  [unwired: 1 in]
            n192 = case shown="True" "Save vis" {
              tunnel: w391 -> [w444 w458]
              tunnel: [w444 w457] -> w395
              tunnel: w390 -> [w443 w456]
              tunnel: [w443 w455] -> w394
              tunnel: w363 -> [_ w446]
              tunnel: w362 -> [_ w449]
              tunnel: w367 -> [_ w448]
              tunnel: w366 -> [_ w447]
              tunnel: w361 -> [_ w445]
              frame False {
              }
              frame True {
                # "Save the data"
                n193 = local read "tdms error out"() -> (w450:errorcluster)
                n194 = local read "tdms file out"() -> (w451:refnum<k34>)
                n195 = case shown="\"Continous Aquisition\", Default" "Mode" {
                  tunnel: w458 -> [w471 w495 w545]
                  tunnel: [w471 w494 w544] -> w457
                  tunnel: w456 -> [w470 w493 w543]
                  tunnel: [w470 w492 w542] -> w455
                  tunnel: w447 -> [_ w490 w540]
                  tunnel: w445 -> [w459 w489 w539]
                  tunnel: w448 -> [_ w488 w532]
                  tunnel: w449 -> [w469 w487 w538]
                  tunnel: w446 -> [w460 w486 w537]
                  tunnel: [w466 w485 w536] -> w453
                  tunnel: [w465 w484 w535] -> w452
                  tunnel: w451 -> [w468 w483 w534]
                  tunnel: w450 -> [w467 w482 w533]
                  tunnel: w445 -> [_ w481 w528]
                  frame "Continous Aquisition", Default {
                    n196 = Quotient & Remainder(x=w459, y="Vis every x aquisition") -> (x-y*floor(x/y)=w463:i32)  [unwired: 1 out]
                    n197 = Equal To 0?(x=w463) -> (x = 0?=w462:bool)
                    n198 = case shown="True" w462 {
                      tunnel: w469 -> [_ w480]
                      tunnel: w468 -> [w473 w479]
                      tunnel: w467 -> [w472 w478]
                      tunnel: [w473 w477] -> w466
                      tunnel: [w472 w476] -> w465
                      tunnel: w460 -> [_ w475]
                      tunnel: w459 -> [_ w474]
                      frame False {
                      }
                      frame True {
                        n199 = call "Writedata_spectra_normonly.vi"("tdms file in"=w479, "Aquisition number"=w474, "Norm Visible Intensity"=w475, "tdms error in"=w478, "Params"=w480) -> ("tdms file out"=w477:refnum<k34>, "tdms error out"=w476:errorcluster)
                      }
                    }
                    n200 = Increment(x=w459) -> (x+1=w461:i32)
                    n201 = local write "vis aq #"(w461) -> ()
                  }
                  frame "Single Aquisition" {
                    # "last iteration?"
                    n202 = call "Writedata_spectra_normonly.vi"("tdms file in"=w483, "Aquisition number"=w481, "Norm Visible Intensity"=w486, "tdms error in"=w482, "Params"=w487) -> ("tdms file out"=w485:refnum<k34>, "tdms error out"=w484:errorcluster)
                    n203 = local read "set vis aq"() -> (w496:i32)
                    n204 = local read "Autoswitch"() -> (w491:bool)
                    n205 = Greater Or Equal?(x=w489, y=w496) -> (x >= y?=w497:bool)
                    n206 = case shown="True" w497 {
                      tunnel: w495 -> [w501 w508]
                      tunnel: w490 -> [_ w509]
                      tunnel: [w501 w507] -> w494
                      tunnel: w493 -> [w500 w506]
                      tunnel: [w500 w505] -> w492
                      tunnel: w489 -> [w498 _]
                      tunnel: w491 -> [_ w503]
                      tunnel: w488 -> [_ w502]
                      frame False {
                        n207 = Increment(x=w498) -> (x+1=w499:i32)
                        n208 = local write "vis aq #"(w499) -> ()
                      }
                      frame True {
                        n209 = Get Date/Time In Seconds() -> (seconds since 1Jan1904=w504:timestamp)
                        n210 = case shown="True" w503 {
                          tunnel: w509 -> [_ w519]
                          tunnel: w508 -> [w511 w518]
                          tunnel: [w511 w517] -> w507
                          tunnel: w506 -> [w510 w516]
                          tunnel: [w510 w515] -> w505
                          tunnel: w504 -> [_ w514]
                          tunnel: w502 -> [_ w513]
                          frame False {
                            n211 = local write "Save vis"(FALSE ("Save Data")) -> ()
                          }
                          frame True {
                            # "done switching?"
                            # "tell MP to switch"
                            n212 = Decimal String To Number(string=w519) -> (number=w520:i32)  [unwired: 2 in, 1 out]
                            n213 = while {
                              tunnel: w514 -> [w526]
                              tunnel: w513 -> [w523]
                              stop <- w524 stop-if-true
                              # "wait at least an integration time"
                              n214 = Get Date/Time In Seconds() -> (seconds since 1Jan1904=w527:timestamp)
                              n215 = Subtract(x=w527, y=w526) -> (x-y=w525:dbl)
                              n216 = Divide(x=w523, y=u32 1000) -> (x/y=w521:dbl)
                              n217 = Greater Or Equal?(x=w525, y=w521) -> (x >= y?=w524:bool)
                            }
                            n218 = Send Notification(notification=w520, notifier=w518) -> (notifier out=w517:refnum<notifier>)  [unwired: 1 in, 1 out]
                            n219 = Wait on Notification(notifier=w516) -> (notifier out=w515:refnum<notifier>)  [unwired: 3 in, 3 out]
                          }
                        }
                      }
                    }
                  }
                  frame "Cont switch" {
                    # "last iteration?"
                    n220 = local read "set vis aq"() -> (w531:i32)
                    n221 = call "Writedata_spectra_normonly.vi"("tdms file in"=w534, "Aquisition number"=w528, "Norm Visible Intensity"=w537, "tdms error in"=w533, "Params"=w538) -> ("tdms file out"=w536:refnum<k34>, "tdms error out"=w535:errorcluster)
                    n222 = Quotient & Remainder(x=w532, y=w531) -> (x-y*floor(x/y)=w529:u32)  [unwired: 1 out]
                    n223 = local read "Autoswitch"() -> (w541:bool)
                    n224 = Equal To 0?(x=w529) -> (x = 0?=w530:bool)
                    n225 = case shown="True" w530 {
                      tunnel: w545 -> [w549 w556]
                      tunnel: w540 -> [_ w557]
                      tunnel: [w549 w555] -> w544
                      tunnel: w543 -> [w548 w554]
                      tunnel: [w548 w553] -> w542
                      tunnel: w539 -> [w546 _]
                      tunnel: w541 -> [_ w551]
                      tunnel: w532 -> [_ w550]
                      frame False {
                        n226 = Increment(x=w546) -> (x+1=w547:i32)
                        n227 = local write "vis aq #"(w547) -> ()
                      }
                      frame True {
                        n228 = Get Date/Time In Seconds() -> (seconds since 1Jan1904=w552:timestamp)
                        n229 = case shown="True" w551 {
                          tunnel: w557 -> [_ w567]
                          tunnel: w556 -> [w559 w566]
                          tunnel: [w559 w565] -> w555
                          tunnel: w554 -> [w558 w564]
                          tunnel: [w558 w563] -> w553
                          tunnel: w552 -> [_ w562]
                          tunnel: w550 -> [_ w561]
                          frame False {
                            n230 = local write "Save vis"(FALSE ("Save Data")) -> ()
                          }
                          frame True {
                            # "done switching?"
                            # "tell MP to switch"
                            n231 = Decimal String To Number(string=w567) -> (number=w568:i32)  [unwired: 2 in, 1 out]
                            n232 = while {
                              tunnel: w562 -> [w574]
                              tunnel: w561 -> [w571]
                              stop <- w572 stop-if-true
                              # "wait at least an integration time"
                              n233 = Get Date/Time In Seconds() -> (seconds since 1Jan1904=w575:timestamp)
                              n234 = Subtract(x=w575, y=w574) -> (x-y=w573:dbl)
                              n235 = Divide(x=w571, y=u32 1000) -> (x/y=w569:dbl)
                              n236 = Greater Or Equal?(x=w573, y=w569) -> (x >= y?=w572:bool)
                            }
                            n237 = Send Notification(notification=w568, notifier=w566) -> (notifier out=w565:refnum<notifier>)  [unwired: 1 in, 1 out]
                            n238 = Wait on Notification(notifier=w564) -> (notifier out=w563:refnum<notifier>)  [unwired: 3 in, 3 out]
                          }
                        }
                      }
                    }
                  }
                }
                n239 = local write "tdms error out"(w452) -> ()
                n240 = local write "tdms file out"(w453) -> ()
              }
            }
            n241 = case shown="False" "Reset BG Vis" {
              frame False {
              }
              frame True {
                n242 = local read "Vis background wave"() -> (w432:cluster{dbl[], dbl[]})
                n243 = Unbundle(w432) -> (w426:dbl[], w431:dbl[])
                n244 = Array Size(array=w431) -> (size(s)=w430:i32)
                n245 = Initialize Array(0.0 ("element"), w430) -> (w427:dbl[])
                n246 = Bundle(w426, w427) -> (w428:cluster{dbl[], dbl[]})  [unwired: 1 in]
                n247 = local write "Vis background wave"(w428) -> ()
                n248 = local write "Reset BG Vis"(FALSE ("Reset Background Vis")) -> ()
                "# averages Vis" <- 1 ("# averages")
              }
            }
            n249 = case shown="True" "Aquire BG vis" {
              tunnel: w373 -> [_ w414]
              frame False {
              }
              frame True {
                n250 = local read "# averages Vis"() -> (w412:i32)
                n251 = local read "Vis background wave"() -> (w423:cluster{dbl[], dbl[]})
                n252 = Divide(x=w414, y=w412) -> (x/y=w418:dbl[])
                n253 = Increment(x=w412) -> (x+1=w420:i32)
                n254 = Decrement(x=w412) -> (x-1=w419:i32)
                n255 = Divide(x=w419, y=w412) -> (x/y=w415:dbl)
                n256 = Unbundle(w423) -> (w421:dbl[], w416:dbl[])
                n257 = Multiply(x=w416, y=w415) -> (x*y=w417:dbl[])
                n258 = local write "# averages Vis"(w420) -> ()
                n259 = Add(x=w417, y=w418) -> (x+y=w413:dbl[])
                n260 = Bundle(w421, w413) -> (w422:cluster{dbl[], dbl[]})  [unwired: 1 in]
                n261 = local write "Vis background wave"(w422) -> ()
              }
            }
            n262 = Unbundle By Name(w396) -> ("status"=w392:bool)
            n263 = Not(x=w392) -> (.not. x?=→"Vis Status":bool)
          }
          n264 = Release Notifier(notifier=w333) -> ()  [unwired: 2 in, 3 out]
          n265 = call <instrlib>:"Close.vi"("error in (no error)"=w337, "VISA resource name"=w338) -> ("error out"=w339:errorcluster)  [unwired: 9 out]
          n266 = Release Notifier(notifier=w332) -> ()  [unwired: 2 in, 3 out]
          n267 = Close Reference(reference=w336, error in (no error)=w335) -> (error out=w340:errorcluster)
          n268 = call <vilib>:"Simple Error Handler.vi"("error in (no error)"=w339) -> ()  [unwired: 1 in, 8 out]
          n269 = call <vilib>:"Simple Error Handler.vi"("error in (no error)"=w340) -> ()  [unwired: 1 in, 8 out]
        }
      }
      n270 = case shown="True" "Use MP" {
        tunnel: w122 -> [_ w233]
        tunnel: w121 -> [_ w232]
        tunnel: w120 -> [_ w231]
        frame False {
        }
        frame True {
          # "Multiplexer setup"
          n271 = Unbundle By Name(T7 {"baud rate"=9600, "data bits"=8, "parity"=enum."None", "stop bits"=10, "flow control"=0} ("Serial Settings")) -> ("baud rate"=w228:u32, "data bits"=w227:u16, "parity"=w226:enum16{"None", "Odd", "Even", "Mark", "Space"}, "stop bits"=w225:u16, "flow control"=w224:u16)
          n272 = local read "Multiplexer Response"() -> (w215:string)
          n273 = call-poly "VISA Configure Serial Port"("VISA resource name"="Multiplexer", "baud rate (9600)"=w228, "data bits (8)"=w227, "parity (0:none)"=w226, "stop bits (10: 1 bit)"=w225, "flow control (0:none)"=w224) -> ("VISA resource name out"=w217:refnum<visa-resource-name>, "error out"=w216:errorcluster)  [unwired: 3 in, 5 out]
          n274 = while {
            tunnel: w217 -> [w254]
            tunnel: w216 -> [w253]
            tunnel: [w252] -> w219
            tunnel: [w251] -> w218
            shift-right: [w249] -> _
            shift-left: w215 -> [w250]
            shift-right: [w238] -> w220
            shift-left: w232 -> [w236]
            shift-right: [w239] -> w221
            shift-left: w233 -> [w235]
            shift-right: [w237] -> w222
            shift-left: w231 -> [w234]
            stop <- "Stop" stop-if-true
            # "multiplexer"
            n275 = local read "Save NIR"() -> (w246:bool)
            n276 = local read "Save vis"() -> (w247:bool)
            n277 = Compound Arithmetic op=AND("Autoswitch", w247, w246) -> (w245:bool)
            n278 = case shown="True" w245 {
              selector: w245 -> [w260 w273]
              tunnel: w235 -> [w259 w264]
              tunnel: w236 -> [w258 w274]
              tunnel: "Position" -> [w261 _]
              tunnel: [w261 w272] -> w243
              tunnel: [w260 w273] -> w240
              tunnel: [w259 w263] -> w239
              tunnel: [w258 w271] -> w238
              frame False {
              }
              frame True {
                # "0 NIR\n1 Vis\n2 Both"
                n279 = local read "Use Vis?"() -> (w270:bool)
                n280 = local read "Use NIR?"() -> (w269:bool)
                n281 = Boolean To (0,1)(Boolean=w270) -> (0, 1=w266:i16)
                n282 = And(x=w269, y=w270) -> (x .and. y?=w268:bool)
                n283 = Boolean To (0,1)(Boolean=w268) -> (0, 1=w267:i16)
                n284 = Add(x=w267, y=w266) -> (x+y=w265:i16)
                n285 = case shown="2" w265 {
                  tunnel: w274 -> [w278 w282 w284]
                  tunnel: [w277 w282 w283] -> w271
                  tunnel: w264 -> [w276 w281 w287]
                  tunnel: [w276 w280 w286] -> w263
                  tunnel: [w275 w279 w285] -> w262
                  frame 0, Default {
                    n286 = Wait on Notification(notifier=w278) -> (notifier out=w277:refnum<notifier>, notification=w275:i32)  [unwired: 3 in, 2 out]
                  }
                  frame 1 {
                    n287 = Wait on Notification(notifier=w281) -> (notifier out=w280:refnum<notifier>, notification=w279:i32)  [unwired: 3 in, 2 out]
                  }
                  frame 2 {
                    n288 = Wait on Notification(notifier=w287) -> (notifier out=w286:refnum<notifier>, notification=w285:i32)  [unwired: 3 in, 2 out]
                    n289 = Wait on Notification(notifier=w284) -> (notifier out=w283:refnum<notifier>)  [unwired: 3 in, 3 out]
                  }
                }
                n290 = case shown="1" w262 {
                  tunnel: [1 0] -> w272
                  frame 0, Default {
                    "MP0 obtained" <- TRUE ("MP0 obtained")
                  }
                  frame 1 {
                    "MP1 obtained" <- TRUE ("MP1 obtained")
                  }
                }
              }
            }
            n291 = Wait (ms)(milliseconds to wait=u32 250 ("Delay (ms)")) -> ()  [unwired: 1 out]
            n292 = Or(x=w240, y="Send to multiplexer") -> (x .or. y?=w242:bool)
            n293 = case shown="True" w242 {
              tunnel: w243 -> [_ w306]
              tunnel: "Multiplexer Command" -> [_ w305]
              tunnel: w254 -> [w295 w304]
              tunnel: w253 -> [w294 w303]
              tunnel: [w295 w297] -> w252
              tunnel: [w294 w302] -> w251
              tunnel: [w293 w296] -> w249
              tunnel: w250 -> [w293 _]
              tunnel: w240 -> [_ w300]
              tunnel: w234 -> [w292 w299]
              tunnel: [w292 w298] -> w237
              frame False {
              }
              frame True {
                n294 = call "Multiplexer_sendsubvi.vi"("error in (no error)"=w303, "Position"=w306, "Enum"=w305, "VISA resource name"=w304) -> ("error out"=w302:errorcluster, "Response"=w296:string, "VISA resource name out"=w297:refnum<visa-resource-name>)
                n295 = local write "Send to multiplexer"(FALSE ("Send to multiplexer")) -> ()
                n296 = case shown="True" w300 {
                  tunnel: w299 -> [w307 w311]
                  tunnel: [w307 w309] -> w298
                  tunnel: w296 -> [_ _]
                  frame False {
                  }
                  frame True {
                    n297 = Send Notification(notification=TRUE, notifier=w311) -> (notifier out=w309:refnum<notifier>)  [unwired: 1 in, 1 out]
                    n298 = local read "Mode"() -> (w308:T5)
                    n299 = case shown="\"Continous Aquisition\"" w308 {
                      frame "Single Aquisition" {
                        w312 = 1
                        n300 = local read "MP0 obtained"() -> (w314:bool)
                        n301 = local read "MP1 obtained"() -> (w315:bool)
                        n302 = local write "NIR aq #"(w312) -> ()
                        n303 = local write "vis aq #"(w312) -> ()
                        n304 = And(x=w314, y=w315) -> (x .and. y?=w313:bool)
                        n305 = case shown="True" w313 {
                          frame False {
                          }
                          frame True {
                            n306 = local write "Save NIR"(FALSE ("Save Data NIR")) -> ()
                            n307 = local write "Save vis"(FALSE ("Save data vis")) -> ()
                          }
                        }
                      }
                      frame "Cont switch" {
                        n308 = local read "NIR aq #"() -> (w319:i32)
                        n309 = local read "vis aq #"() -> (w318:i32)
                        n310 = local read "MP0 obtained"() -> (w323:bool)
                        n311 = local read "MP1 obtained"() -> (w324:bool)
                        n312 = Increment(x=w319) -> (x+1=w320:i32)
                        n313 = Increment(x=w318) -> (x+1=w321:i32)
                        n314 = And(x=w323, y=w324) -> (x .and. y?=w322:bool)
                        n315 = local write "NIR aq #"(w320) -> ()
                        n316 = local write "vis aq #"(w321) -> ()
                        n317 = case shown="True" w322 {
                          frame False {
                          }
                          frame True {
                            w325 = FALSE
                            n318 = local write "MP0 obtained"(w325) -> ()
                            n319 = local write "MP1 obtained"(w325) -> ()
                          }
                        }
                      }
                      frame "Continous Aquisition" {
                        w326 = 1
                        n320 = local read "MP0 obtained"() -> (w328:bool)
                        n321 = local read "MP1 obtained"() -> (w329:bool)
                        n322 = local write "NIR aq #"(w326) -> ()
                        n323 = local write "vis aq #"(w326) -> ()
                        n324 = And(x=w328, y=w329) -> (x .and. y?=w327:bool)
                        n325 = case shown="True" w327 {
                          frame False {
                          }
                          frame True {
                            n326 = local write "Save NIR"(FALSE ("Save Data NIR")) -> ()
                            n327 = local write "Save vis"(FALSE ("Save data vis")) -> ()
                          }
                        }
                      }
                    }
                  }
                }
              }
            }
            "Multiplexer Response" <- w249
          }
          n328 = VISA Close(VISA resource name=w219, error in (no error)=w218) -> (error out=w223:errorcluster)
          n329 = Release Notifier(notifier=w221) -> ()  [unwired: 2 in, 3 out]
          n330 = Release Notifier(notifier=w220) -> ()  [unwired: 2 in, 3 out]
          n331 = Release Notifier(notifier=w222) -> ()  [unwired: 2 in, 3 out]
          n332 = call <vilib>:"Simple Error Handler.vi"("error in (no error)"=w223) -> ()  [unwired: 1 in, 8 out]
        }
      }
      n333 = while {
        stop <- w173 stop-if-true
        w132 = string[] ["Bandwidth 1-2", "Bandwidth 2-3", "Bandwidth 1-3"]
        w169 = "Temp"
        w137 = "Temperature"
        n334 = local read "Norm Visible Intensity"() -> (w199:cluster{dbl[], dbl[]})
        n335 = local read "Norm NIR Intensity"() -> (w154:cluster{dbl[], dbl[]})
        n336 = Divide(x="Bandwidth 2", y=2) -> (x/y=w194:dbl)
        n337 = Divide(x="Bandwidth 3", y=2) -> (x/y=w195:dbl)
        n338 = Unbundle(w199) -> (w152:dbl[], w149:dbl[])
        n339 = Unbundle(w154) -> (w153:dbl[], w150:dbl[])
        n340 = Array Size(array=w152) -> (size(s)=w151:i32)
        n341 = Divide(x="Bandwidth 1", y=2) -> (x/y=w178:dbl)
        n342 = Array Size(array=w149) -> (size(s)=w148:i32)
        n343 = Insert Into Array(array=w152, index=w151, new element=w153) -> (w147:dbl[])
        n344 = Insert Into Array(array=w149, index=w148, new element=w150) -> (w146:dbl[])
        n345 = call "Search 1D Array for Nearest LV2012 NIVerified.vi"("desired element"="Wavelength 1", "1D Array"=w147) -> ("closest index"=w176:i32, "closest element"=w174:dbl)  [unwired: 8 in]
        n346 = call "Search 1D Array for Nearest LV2012 NIVerified.vi"("desired element"="Wavelength 3", "1D Array"=w147) -> ("closest index"=w179:i32)  [unwired: 8 in, 1 out]
        n347 = call "Search 1D Array for Nearest LV2012 NIVerified.vi"("desired element"="Wavelength 2", "1D Array"=w147) -> ("closest index"=w177:i32)  [unwired: 8 in, 1 out]
        n348 = Subtract(x=w176, y=w178) -> (x-y=w182:dbl)
        n349 = Subtract(x=w177, y=w194) -> (x-y=w181:dbl)
        n350 = Subtract(x=w179, y=w195) -> (x-y=w180:dbl)
        n351 = Array Subset(array=w146, index=w182, length="Bandwidth 1") -> (w185:dbl[])
        n352 = Array Subset(array=w146, index=w181, length="Bandwidth 2") -> (w184:dbl[])
        n353 = Array Subset(array=w146, index=w180, length="Bandwidth 3") -> (w183:dbl[])
        n354 = call <vilib>:"Std Deviation and Variance.vi"("X"=w184) -> ("mean"=w187:dbl, "standard deviation"=→"stddev 2":dbl)  [unwired: 1 in, 1 out]
        "Mean 2" <- w187
        n355 = call <vilib>:"Std Deviation and Variance.vi"("X"=w183) -> ("mean"=w188:dbl, "standard deviation"=→"stddev 3":dbl)  [unwired: 1 in, 1 out]
        "Mean 3" <- w188
        n356 = call <vilib>:"Std Deviation and Variance.vi"("X"=w185) -> ("mean"=w186:dbl, "standard deviation"=→"stddev":dbl)  [unwired: 1 in, 1 out]
        "Mean" <- w186
        n357 = Number To Decimal String(number="Wavelength 1") -> (decimal integer string=w160:string)  [unwired: 1 in]
        n358 = Number To Decimal String(number="Wavelength 2") -> (decimal integer string=w145:string)  [unwired: 1 in]
        n359 = Number To Decimal String(number="Wavelength 3") -> (decimal integer string=w158:string)  [unwired: 1 in]
        n360 = call "2_color_temp_subVI_discrete.vi"("E1 2"=w187, "E1"=w186, "In_WL1 2"="Wavelength 2", "In_WL1"=w174) -> ("FT"=w172:dbl)  [unwired: 7 in]
        "Temp 1-2" <- w172
        n361 = call "2_color_temp_subVI_discrete.vi"("E1 2"=w188, "E1"=w186, "In_WL1 2"="Wavelength 3", "In_WL1"="Wavelength 1") -> ("FT"=w171:dbl)  [unwired: 7 in]
        "Temp 1-3" <- w171
        n362 = call "2_color_temp_subVI_discrete.vi"("E1 2"=w188, "E1"=w187, "In_WL1 2"="Wavelength 3", "In_WL1"="Wavelength 2") -> ("FT"=w170:dbl)  [unwired: 7 in]
        "Temp 2-3" <- w170
        n363 = Concatenate Strings(w160, "-" ("string"), w145) -> (w157:string)
        n364 = Concatenate Strings(w145, "-" ("string"), w158) -> (w155:string)
        n365 = Concatenate Strings(w160, "-" ("string"), w158) -> (w156:string)
        n366 = Build Array(w172) -> (w198:dbl[])
        n367 = Build Array(w171) -> (w197:dbl[])
        n368 = Build Array(w170) -> (w196:dbl[])
        n369 = local read "tdms error out"() -> (w206:errorcluster)
        n370 = local read "tdms file out"() -> (w205:refnum<k34>)
        n371 = Concatenate Strings(w169, w157) -> (w168:string)
        n372 = Concatenate Strings(w169, w156) -> (w167:string)
        n373 = Concatenate Strings(w169, w155) -> (w166:string)
        n374 = Build Array(w168, w167, w166) -> (w131:string[])
        n375 = Build Array(w198, w197, w196) -> (w133:dbl[][])
        n376 = TDMS Write(0:w205, 5:w137, 7:w131, 9:w133, 11:w206) -> (4:w203:refnum<k34>, 15:w204:errorcluster)  [unwired: 1 in, 2 out]
        n377 = Build Array("Bandwidth 1", "Bandwidth 2", "Bandwidth 3") -> (w134:i32[])
        n378 = Get Date/Time In Seconds() -> (seconds since 1Jan1904=w201:timestamp)
        n379 = Build Array(w201) -> (w200:timestamp[])
        n380 = TDMS Write(0:w203, 5:w137, 7:"Time" ("channel name(s) in (Untitled)"), 9:w200, 11:w204) -> (4:w140:refnum<k34>, 15:w136:errorcluster)  [unwired: 1 in, 2 out]
        n381 = local read "Stop"() -> (w173:bool)
        n382 = for {
          tunnel: w137 -> [w211]
          tunnel: w134 -> [w209] mode=indexing
          tunnel: w132 -> [w208] mode=indexing
          shift-right: [w213] -> w139
          shift-left: w140 -> [w214]
          shift-right: [w212] -> w138
          shift-left: w136 -> [w210]
          tunnel: w131 -> [w207] mode=indexing
          n383 = TDMS Set Properties(5:w209, 7:w208, 8:w210, 9:w207, 10:w211, 11:w214) -> (0:w212:errorcluster, 3:w213:refnum<k34>)  [unwired: 2 out]
        }
        n384 = Wait (ms)(milliseconds to wait=u32 100) -> ()  [unwired: 1 out]
        n385 = local read "NIR Data"() -> (w126:T2)
        n386 = local read "Vis Data"() -> (w125:T3)
        n387 = local write "tdms error out"(w138) -> ()
        n388 = local write "tdms file out"(w139) -> ()
        n389 = Get Date/Time In Seconds() -> (seconds since 1Jan1904=w135:timestamp)
        n390 = Bundle(cluster=T6 {"Bandwidth"=[], "Bandwidth labels"=[], "Color Temperatures"=[], "Wavelength labels"=[], "seconds since 1Jan1904"=timestamp(0 s since 1904-01-01)}, "Bandwidth"=w134, "Bandwidth labels"=w132, "Color Temperatures"=w133, "Wavelength labels"=w131, "seconds since 1Jan1904"=w135) -> (w129:T6)
        n391 = Bundle(cluster=T1 {"Temperature Data"={"Bandwidth"=[], "Bandwidth labels"=[], "Color Temperatures"=[], "Wavelength labels"=[], "seconds since 1Jan1904"=timestamp(0 s since 1904-01-01)}, "Vis Data"={{"visible wl array"=[], []}, {"Vis or NIR"="", "Multiplexer Response"="", "Wavelength Difference Vis (nm)"=0.0, "Vis Integration Time (ms)"=0, "Normalization path"=path "", "Vis background wave"={[], []}}}, "NIR Data"={{"NIR wl array"=[], []}, {"Vis or NIR"="", "Multiplexer Response"="", "NIR Integration Time (ms)"=0, "Wavelength Difference NIR (nm) "=0.0, "Normalization path"=path "", "NIR background wave"={[], []}}}}, "Temperature Data"=w129, "Vis Data"=w125, "NIR Data"=w126) -> (w127:T1)
        n392 = property on="output cluster" class="Clust (strict)"("Val(Sgnl)"=w127) -> ()  [unwired: 2 in, 2 out]
      }
      n393 = while {
        tunnel: w112 -> [w815]
        tunnel: w111 -> [w814]
        tunnel: w110 -> [w813]
        stop <- w835 stop-if-true
        n394 = local read "Save NIR"() -> (w833:bool)
        n395 = local read "set IR aq"() -> (w830:i32)
        n396 = local read "NIR aq #"() -> (w829:i32)
        n397 = local read "Save vis"() -> (w834:bool)
        n398 = local read "set vis aq"() -> (w831:i32)
        n399 = local read "vis aq #"() -> (w832:i32)
        n400 = event shown="[5] \"base path\", \"Filename\": Value Change" {
          selector: _ -> [_ _ _ _ _ _]
          dyn-events: _ -> [_ _ _ _ _ _]
          timeout: 10 -> [_ _ _ _ _ _]
          tunnel: w815 -> [_ _ _ w849 _ _]
          tunnel: w814 -> [_ _ _ w848 _ _]
          tunnel: w813 -> [_ _ _ w847 _ _]
          event Timeout {
            n401 = event-data() -> ()  [unwired: 1 in, 3 out]
          }
          event "Vis Integration Time (ms)": Value Change {
            n402 = event-data() -> ()  [unwired: 1 in, 6 out]
            "Chg vis time" <- TRUE ("Change NIR time")
          }
          event "Stop aquisition": Mouse Down {
            n403 = event-data() -> ()  [unwired: 1 in, 8 out]
            n404 = local write "Save NIR"(FALSE ("Save Data NIR")) -> ()
            n405 = local write "Save vis"(FALSE ("Save data vis")) -> ()
          }
          event "Clear": Mouse Down {
            n406 = event-data() -> ()  [unwired: 1 in, 8 out]
            n407 = Cancel Notification(0:w848) -> ()  [unwired: 1 in, 3 out]
            n408 = Cancel Notification(0:w849) -> ()  [unwired: 1 in, 3 out]
            n409 = Cancel Notification(0:w847) -> ()  [unwired: 1 in, 3 out]
          }
          event "NIR Integration Time (ms)": Value Change {
            n410 = event-data() -> ()  [unwired: 1 in, 6 out]
            "Change NIR time" <- TRUE ("Change NIR time")
          }
          event "base path", "Filename": Value Change {
            n411 = event-data() -> ()  [unwired: 1 in, 6 out]
            n412 = flat-sequence {
              frame #0 {
                n413 = local read "tdms error out"() -> (w852:errorcluster)
                n414 = local read "tdms file out"() -> (w851:refnum<k34>)
                n415 = TDMS Close(8:w852, 11:w851) -> ()  [unwired: 2 out]
              }
              frame #1 {
                w865 = "Wavelength" ("group name in (Untitled)")
                n416 = local read "Filename"() -> (w855:string)
                n417 = local read "base path"() -> (w854:path)
                n418 = call "GenerateFilepathLA1.vi"("Auto Date folder"=TRUE, "Filename"=w855, "base path"=w854) -> ("Numeric"=w856:i32, "file path"=w857:path)  [unwired: 1 in, 1 out]
                n419 = local write "file path"(w857) -> ()
                n420 = TDMS Open(10:w856, 11:w857) -> (0:w862:errorcluster, 3:w863:refnum<k34>)  [unwired: 5 in]
                n421 = local read "NIR wl array"() -> (w858:dbl[])
                n422 = TDMS Write(0:w863, 5:w865, 7:"NIR" ("group name in (Untitled)"), 9:w858, 11:w862) -> (4:w867:refnum<k34>, 15:w868:errorcluster)  [unwired: 1 in, 2 out]
                n423 = local read "visible wl array"() -> (w859:dbl[])
                n424 = TDMS Write(0:w867, 5:w865, 7:"Visible" ("group name in (Untitled)"), 9:w859, 11:w868) -> (4:w861:refnum<k34>, 15:w860:errorcluster)  [unwired: 1 in, 2 out]
                n425 = local write "tdms error out"(w860) -> ()
                n426 = local write "tdms file out"(w861) -> ()
              }
            }
          }
        }
        n427 = Wait (ms)(milliseconds to wait=u32 250) -> ()  [unwired: 1 out]
        n428 = Not(x=w834) -> (.not. x?=w828:bool)
        n429 = Not(x=w833) -> (.not. x?=w827:bool)
        n430 = Greater Or Equal?(x=w829, y=w830) -> (x >= y?=w825:bool)
        n431 = Greater Or Equal?(x=w832, y=w831) -> (x >= y?=w826:bool)
        n432 = Compound Arithmetic op=AND(w828, w827, w826, w825) -> (w823:bool)
        n433 = Or(x="reset aquisitions", y=w823) -> (x .or. y?=w822:bool)
        n434 = local read "file path"() -> (w821:path)
        n435 = case shown="True" w822 {
          frame False {
          }
          frame True {
            w881 = 1
            n436 = local write "reset aquisitions"(FALSE ("reset aquisitions")) -> ()
            n437 = local write "NIR aq #"(w881) -> ()
            n438 = local write "vis aq #"(w881) -> ()
          }
        }
        n439 = File/Directory Info(path=w821) -> (size=w817:i64, error out=w819:errorcluster)  [unwired: 1 in, 5 out]
        "file size" <- w817
        n440 = call <vilib>:"Simple Error Handler.vi"("error in (no error)"=w819) -> ()  [unwired: 1 in, 8 out]
        n441 = local read "Stop"() -> (w835:bool)
        n442 = case shown="True" "save both" {
          tunnel: w817 -> [_ w872]
          frame False {
          }
          frame True {
            n443 = Greater?(x=w872, y=i64 0) -> (0:w870:bool)
            n444 = case shown="True" w870 {
              tunnel: [TRUE w879] -> w869
              frame False {
              }
              frame True {
                n445 = Two Button Dialog(message="Saving into existing file, continue?  ") -> (T button?=w879:bool)  [unwired: 2 in]
              }
            }
            n446 = case shown="True" w869 {
              frame False {
                n447 = local write "save both"(FALSE ("save both")) -> ()
              }
              frame True {
                w874 = FALSE ("save both")
                n448 = local write "Save NIR"(TRUE ("Save Data NIR")) -> ()
                n449 = local write "Save vis"(TRUE ("Save data vis")) -> ()
                n450 = local write "save both"(FALSE ("save both")) -> ()
                n451 = local write "MP0 obtained"(w874) -> ()
                n452 = local write "MP1 obtained"(w874) -> ()
              }
            }
          }
        }
        n453 = case shown="False" "Cal params" {
          frame False {
          }
          frame True {
            n454 = local write "Cal params"(FALSE ("Cal params")) -> ()
            n455 = local write "NIR Integration Time (ms)"(u32 50 ("NIR Integration Time (ms)")) -> ()
            n456 = local write "Vis Integration Time (ms)"(u32 1000 ("Vis Integration Time (ms)")) -> ()
            n457 = local write "set vis aq"(20 ("set vis aq")) -> ()
            n458 = local write "set IR aq"(200 ("set IR aq")) -> ()
            n459 = local write "Send to multiplexer"(TRUE ("Send to multiplexer")) -> ()
            n460 = local write "Position"(0 ("Position")) -> ()
          }
        }
      }
    }
    frame #2 {
      n461 = local read "tdms error out"() -> (w886:errorcluster)
      n462 = local read "tdms file out"() -> (w887:refnum<k34>)
      n463 = local write "Save NIR"(FALSE ("Save Data NIR")) -> ()
      n464 = local write "Save vis"(FALSE ("Save data vis")) -> ()
      n465 = local write "Stop"(FALSE ("Stop")) -> ()
      n466 = TDMS Close(8:w886, 11:w887) -> (0:w885:errorcluster)  [unwired: 1 out]
      n467 = call <vilib>:"Simple Error Handler.vi"("error in (no error)"=w885) -> ()  [unwired: 1 in, 8 out]
    }
  }
